vi "Defect Buddy.vi"() -> ()   [LabVIEW 2010]
uses:
  <vilib>/addons/database/Connection.llb/Conn ObjectReference.ctl
  <vilib>/addons/database/_DB Variant To Data/Database Variant To Data.xnode
  <vilib>/addons/database/Connection.llb/DB Tools Open Connec (Path).vi
  <vilib>/addons/database/Connection.llb/Conn Execute.vi
  <vilib>/addons/database/Recordset.llb/Rec Fetch Recordset Data (R).vi
  <vilib>/addons/database/Recordset.llb/Rec Destroy - Connection.vi
  <vilib>/Utility/file.llb/Write To Spreadsheet File (string).vi
  <vilib>/addons/database/NI_Database_API.lvlib
  <vilib>/picture/3D Picture Control/NI_3D Picture Control.lvlib
panel:
  out "Plot Names":string[][](array[string])
  out "Separate Defects":cluster{i32, i32}[](array[cluster])
  in  "Bound Pairs":T1(array[cluster])
  out "Array 2":T2(array[cluster])
  out "Array":string[][](array[string])
  out "spreadsheet string":string
  in  "Volumes":dbl[](array[numeric])=[5230.5515143, 4360.60278, 2309.371815, 7792.576126]
  in  "Markov-Payne Correction":bool=TRUE
  out "Loaded Structure":T3={"Structure Name"="Batch6_3+111 Quasi-Bulk", "Lattice vector a"=[9.1641, 0.0, 0.0], "Lattice vector b"=[0.0, 7.93635, 0.0], "Lattice vector c"=[0.0, 0.0, 53.7091], "Atoms Array"=[{"Atom Name"="", "Positions (Direct)"=[[0.036896, 0.129554, 0.035254], [0.536896, 0.129554, 0.035254], [0.286896, 0.629554, 0.035254], [0.786896, 0.629554, 0.035254], [0.285415, 0.295133, 0.107673], [0.785415, 0.295133, 0.107673], [0.035415, 0.795133, 0.107673], [0.535415, 0.795133, 0.107673], [0.033615, 0.463308, 0.180101], [0.533615, 0.463308, 0.180101], [0.283615, 0.963308, 0.180101], [0.783615, 0.963308, 0.180101], [0.030844, 0.131453, 0.252535], [0.530844, 0.131453, 0.252535], [0.280844, 0.631453, 0.252535], [0.780844, 0.631453, 0.252535], [0.278379, 0.302058, 0.324923], [0.778379, 0.302058, 0.324923], [0.028379, 0.802058, 0.324923], [0.528379, 0.802058, 0.324923], [0.031198, 0.471844, 0.397363], [0.531198, 0.471844, 0.397363], [0.281198, 0.971844, 0.397363], [0.781198, 0.971844, 0.397363], [0.03247, 0.140643, 0.469814], [0.53247, 0.140643, 0.469814], [0.28247, 0.640643, 0.469814], [0.78247, 0.640643, 0.469814], [0.284308, 0.303948, 0.542263], [0.784308, 0.303948, 0.542263], [0.034308, 0.803948, 0.542263], [0.534308, 0.803948, 0.542263], [0.035944, 0.468219, 0.614701], [0.535944, 0.468219, 0.614701], [0.285944, 0.968219, 0.614701], [0.785944, 0.968219, 0.614701], [0.037813, 0.131858, 0.687216], [0.537813, 0.131858, 0.687216], [0.787813, 0.631858, 0.687216], [0.287813, 0.631858, 0.687216], [0.038238, 0.463759, 0.759817], [0.538238, 0.463759, 0.759817], [0.288238, 0.963758, 0.759817], [0.788238, 0.963758, 0.759817], [0.038639, 0.130134, 0.831025], [0.538639, 0.130134, 0.831025], [0.288639, 0.630134, 0.831025], [0.788639, 0.630134, 0.831025], [0.285712, 0.295024, 0.89873], [0.785712, 0.295024, 0.89873], [0.035712, 0.795024, 0.89873], [0.535712, 0.795024, 0.89873], [0.032596, 0.464879, 0.966384], [0.532596, 0.464879, 0.966384], [0.282596, 0.964879, 0.966384], [0.782596, 0.964879, 0.966384]], "Positions (Cartesian)"=[[0.33811863359999994, 1.0281858879, 1.8934606114], [4.9201686336, 1.0281858879, 1.8934606114], [2.6291436335999996, 4.9963608879, 1.8934606114], [7.2111936336, 4.9963608879, 1.8934606114], [2.6155716014999997, 2.34227878455, 5.7830199243000004], [7.197621601499999, 2.34227878455, 5.7830199243000004], [0.3245466015, 6.31045378455, 5.7830199243000004], [4.9065966014999995, 6.31045378455, 5.7830199243000004], [0.30805122149999997, 3.6769744458, 9.673062619100001], [4.890101221499999, 3.6769744458, 9.673062619100001], [2.5990762215, 7.6451494458, 9.673062619100001], [7.1811262215, 7.6451494458, 9.673062619100001], [0.2826575004, 1.04325701655, 13.5634275685], [4.8647075004, 1.04325701655, 13.5634275685], [2.5736825004, 5.011432016550001, 13.5634275685], [7.155732500399999, 5.011432016550001, 13.5634275685], [2.5510929938999998, 2.3972380083, 17.4513218993], [7.1331429939, 2.3972380083, 17.4513218993], [0.2600679939, 6.3654130083, 17.4513218993], [4.8421179939000005, 6.3654130083, 17.4513218993], [0.28590159179999997, 3.7447191294, 21.3420091033], [4.867951591799999, 3.7447191294, 21.3420091033], [2.5769265918, 7.7128941294, 21.3420091033], [7.158976591799999, 7.7128941294, 21.3420091033], [0.29755832699999996, 1.11619207305, 25.2332871074], [4.879608327, 1.11619207305, 25.2332871074], [2.588583327, 5.08436707305, 25.2332871074], [7.170633327, 5.08436707305, 25.2332871074], [2.6054269428, 2.4122377098, 29.124457693300002], [7.1874769428, 2.4122377098, 29.124457693300002], [0.31440194279999994, 6.3804127098, 29.124457693300002], [4.8964519428, 6.3804127098, 29.124457693300002], [0.32939441039999995, 3.71594986065, 33.0150374791], [4.9114444104, 3.71594986065, 33.0150374791], [2.6204194104, 7.684124860650001, 33.0150374791], [7.202469410399999, 7.684124860650001, 33.0150374791], [0.3465221133, 1.0464712383, 36.909752865600005], [4.9285721133, 1.0464712383, 36.909752865600005], [7.2195971133, 5.0146462383, 36.909752865600005], [2.6375471132999997, 5.0146462383, 36.909752865600005], [0.3504168558, 3.6805537396499997, 40.809087234699994], [4.9324668557999995, 3.6805537396499997, 40.809087234699994], [2.6414418557999997, 7.6487208033, 40.809087234699994], [7.2234918558, 7.6487208033, 40.809087234699994], [0.35409165989999997, 1.0327889709, 44.6336048275], [4.9361416599, 1.0327889709, 44.6336048275], [2.6451166599, 5.0009639709, 44.6336048275], [7.227166659899999, 5.0009639709, 44.6336048275], [2.6182933392, 2.3414137224, 48.269979443000004], [7.200343339199999, 2.3414137224, 48.269979443000004], [0.3272683392, 6.3095887224, 48.269979443000004], [4.9093183391999995, 6.3095887224, 48.269979443000004], [0.29871300359999997, 3.6894424516499997, 51.9036148944], [4.880763003599999, 3.6894424516499997, 51.9036148944], [2.5897380036, 7.65761745165, 51.9036148944], [7.171788003599999, 7.65761745165, 51.9036148944]]}, {"Atom Name"="", "Positions (Direct)"=[[0.286795, 0.296109, 0.054458], [0.786795, 0.296109, 0.054458], [0.036795, 0.796109, 0.054458], [0.536795, 0.796109, 0.054458], [0.035258, 0.462031, 0.126878], [0.535258, 0.462031, 0.126878], [0.285258, 0.962031, 0.126878], [0.785258, 0.962031, 0.126878], [0.033445, 0.130094, 0.199309], [0.533445, 0.130094, 0.199309], [0.283445, 0.630094, 0.199309], [0.783445, 0.630094, 0.199309], [0.280766, 0.298203, 0.27171], [0.780766, 0.298203, 0.27171], [0.030766, 0.798203, 0.27171], [0.530766, 0.798203, 0.27171], [0.028505, 0.468822, 0.344121], [0.528505, 0.468822, 0.344121], [0.278505, 0.968822, 0.344121], [0.778505, 0.968822, 0.344121], [0.03126, 0.138635, 0.416572], [0.53126, 0.138635, 0.416572], [0.28126, 0.638635, 0.416572], [0.78126, 0.638635, 0.416572], [0.282556, 0.307128, 0.489026], [0.782556, 0.307128, 0.489026], [0.032556, 0.807128, 0.489026], [0.532556, 0.807128, 0.489026], [0.034374, 0.470438, 0.56147], [0.534374, 0.470438, 0.56147], [0.284374, 0.970438, 0.56147], [0.784374, 0.970438, 0.56147], [0.035964, 0.134698, 0.633895], [0.535964, 0.134698, 0.633895], [0.285964, 0.634698, 0.633895], [0.785964, 0.634698, 0.633895], [0.037794, 0.465111, 0.706493], [0.537794, 0.465111, 0.706493], [0.787794, 0.965111, 0.706493], [0.287794, 0.965111, 0.706493], [0.038181, 0.130274, 0.779081], [0.538181, 0.130274, 0.779081], [0.288181, 0.630273, 0.779081], [0.788181, 0.630273, 0.779081], [0.288548, 0.296604, 0.847022], [0.788548, 0.296604, 0.847022], [0.038548, 0.796604, 0.847022], [0.538548, 0.796604, 0.847022], [0.035661, 0.461866, 0.914714], [0.535661, 0.461866, 0.914714], [0.285661, 0.961866, 0.914714], [0.785661, 0.961866, 0.914714], [0.032517, 0.131341, 0.982331], [0.532517, 0.131341, 0.982331], [0.282517, 0.631341, 0.982331], [0.782517, 0.631341, 0.982331]], "Positions (Cartesian)"=[[2.6282180595, 2.35002466215, 2.9248901678], [7.2102680595, 2.35002466215, 2.9248901678], [0.3371930595, 6.31819966215, 2.9248901678], [4.9192430595, 6.31819966215, 2.9248901678], [0.32310783779999996, 3.66683972685, 6.814503189799999], [4.9051578378, 3.66683972685, 6.814503189799999], [2.6141328378, 7.63501472685, 6.814503189799999], [7.1961828377999995, 7.63501472685, 6.814503189799999], [0.3064933245, 1.0324715168999998, 10.704707011899998], [4.8885433245, 1.0324715168999998, 10.704707011899998], [2.5975183244999998, 5.000646516900001, 10.704707011899998], [7.179568324499999, 5.000646516900001, 10.704707011899998], [2.5729677006, 2.36664337905, 14.593299561], [7.155017700599999, 2.36664337905, 14.593299561], [0.2819427006, 6.33481837905, 14.593299561], [4.863992700599999, 6.33481837905, 14.593299561], [0.2612226705, 3.7207354797, 18.4824292011], [4.843272670499999, 3.7207354797, 18.4824292011], [2.5522476705, 7.6889104797, 18.4824292011], [7.1342976705, 7.6889104797, 18.4824292011], [0.286469766, 1.1002558822500002, 22.3737072052], [4.8685197659999995, 1.1002558822500002, 22.3737072052], [2.577494766, 5.0684308822499995, 22.3737072052], [7.159544765999999, 5.0684308822499995, 22.3737072052], [2.5893714396, 2.4374753028000002, 26.2651463366], [7.1714214396, 2.4374753028000002, 26.2651463366], [0.2983464396, 6.4056503028, 26.2651463366], [4.8803964396, 6.4056503028, 26.2651463366], [0.3150067734, 3.7335606213, 30.156048377], [4.8970567734, 3.7335606213, 30.156048377], [2.6060317734, 7.7017356213, 30.156048377], [7.1880817733999995, 7.7017356213, 30.156048377], [0.3295776924, 1.0690104723, 34.045929944499996], [4.9116276924, 1.0690104723, 34.045929944499996], [2.6206026924, 5.0371854723, 34.045929944499996], [7.202652692399999, 5.0371854723, 34.045929944499996], [0.3463479954, 3.69128368485, 37.9451031863], [4.928397995399999, 3.69128368485, 37.9451031863], [7.2194229953999995, 7.659458684850001, 37.9451031863], [2.6373729954, 7.659458684850001, 37.9451031863], [0.34989450209999995, 1.0339000599000001, 41.843739337100004], [4.9319445020999995, 1.0339000599000001, 41.843739337100004], [2.6409195021, 5.00206712355, 41.843739337100004], [7.2229695021, 5.00206712355, 41.843739337100004], [2.6442827268, 2.3539531553999997, 45.4927893002], [7.2263327268, 2.3539531553999997, 45.4927893002], [0.35325772679999995, 6.3221281554, 45.4927893002], [4.9353077268, 6.3221281554, 45.4927893002], [0.3268009701, 3.6655302291, 49.1284656974], [4.9088509701000005, 3.6655302291, 49.1284656974], [2.6178259700999997, 7.6337052291, 49.1284656974], [7.1998759701, 7.6337052291, 49.1284656974], [0.29798903969999996, 1.04236814535, 52.760113912099996], [4.8800390397, 1.04236814535, 52.760113912099996], [2.5890140397, 5.010543145350001, 52.760113912099996], [7.1710640397, 5.010543145350001, 52.760113912099996]]}], "# of atoms"=112}
  out "Indicies":cluster{i32, i32}[](array[cluster])
  out "All Hosts and Defects":T4(array[cluster])
  out "Thermodynamic Fermi Level (eV)":dbl
  out "Defects to Bind":i32[](array[numeric])
  in  "Plot Binding Energy":bool
  in  "Calc Thermodynamic Fermi Level":bool
  in  "Thermodynamic Fermi Level":i32
  in  "Color Array Type":T5(ring)=enum."Contrasting Colors"
  in  "Show Charge Transitions":bool=TRUE
  out "connection reference":T6
  in  "Plots Tab":T7(tab)
  in  "Make Awesome Looking":bool
  out "Te Rich Limit":cluster{dbl[], dbl[]}[](graph)
  out "Cd Rich Limit":cluster{"appended array":dbl[], dbl[]}[](graph)
  in  "Chemical Potential":dbl(slide) scale=0.0..1.0
  in  "Chemical Potential 2":dbl(slide)=1.0 scale=0.0..1.0
  in  "Save as a table":bool
  out "Te Rich Limit 2":cluster{dbl[], dbl[]}[](graph)
  out "Cd Rich Limit 2":cluster{"appended array":dbl[], dbl[]}[](graph)
  in  "Chemical Potential 5":dbl(slide) scale=0.0..1.0
  in  "Chemical Potential 3":dbl(slide)=1.0 scale=0.0..1.0
  in  "Save as a table 2":bool
  in  "Binding Energy":bool
  in  "Formation Energy":bool
  in  "Bound Pairs List":i32[](listbox)
  in  "Assign Bound Calculation":bool
  in  "Seperate Defects":i32(listbox)
  in  "Set as seperate defects":bool
  out "Binding Energy":cluster{"Array":dbl[], dbl[]}[](graph)
  in  "Binding Energy Chem Pot":dbl(slide) scale=0.0..1.0
  out "Defect Energy Levels":cluster{dbl[], dbl[]}[](graph)
  in  "Buckets":string[][](array[combo])
  out "Atomic Structure":refnum<vi>(3d-picture)
  in  "Load in VESTA":bool
  in  "Atomic Structures":i32(listbox)
  in  "Options":cluster{"Border?":bool, "Bonds?":bool}
  in  "Atom Size":dbl=0.75
  in  "Plot Atomic Structure":bool
  in  "Scale":dbl(slide)=0.07482993197278912 scale=0.0..0.5
  in  "Setup Camera":bool
  out "Table Control":string[][](table)
  in  "Ignore Location":bool
  in  "Potential Re-alignment":bool
  out "Defects":T8(array[cluster])
  out "Base Object":refnum<vi>
  in  "VBM":dbl=1.79581
  in  "Ignore Incomplete":bool
  in  "Pure Structures with defects":i32[](listbox)
  in  "Related Defects":i32[](listbox)
  in  "UDL":path=path "D:/Ab-initio/VASP Calcs/VASP DB.udl"
  # "Cd Rich"
  # "Te Rich"
  # "Cd Rich"
  # "Te Rich"
  # "p-type"
  # "n-type"
  # "p-type"
  # "n-type"
  # "Cd Rich"
  # "Te Rich"
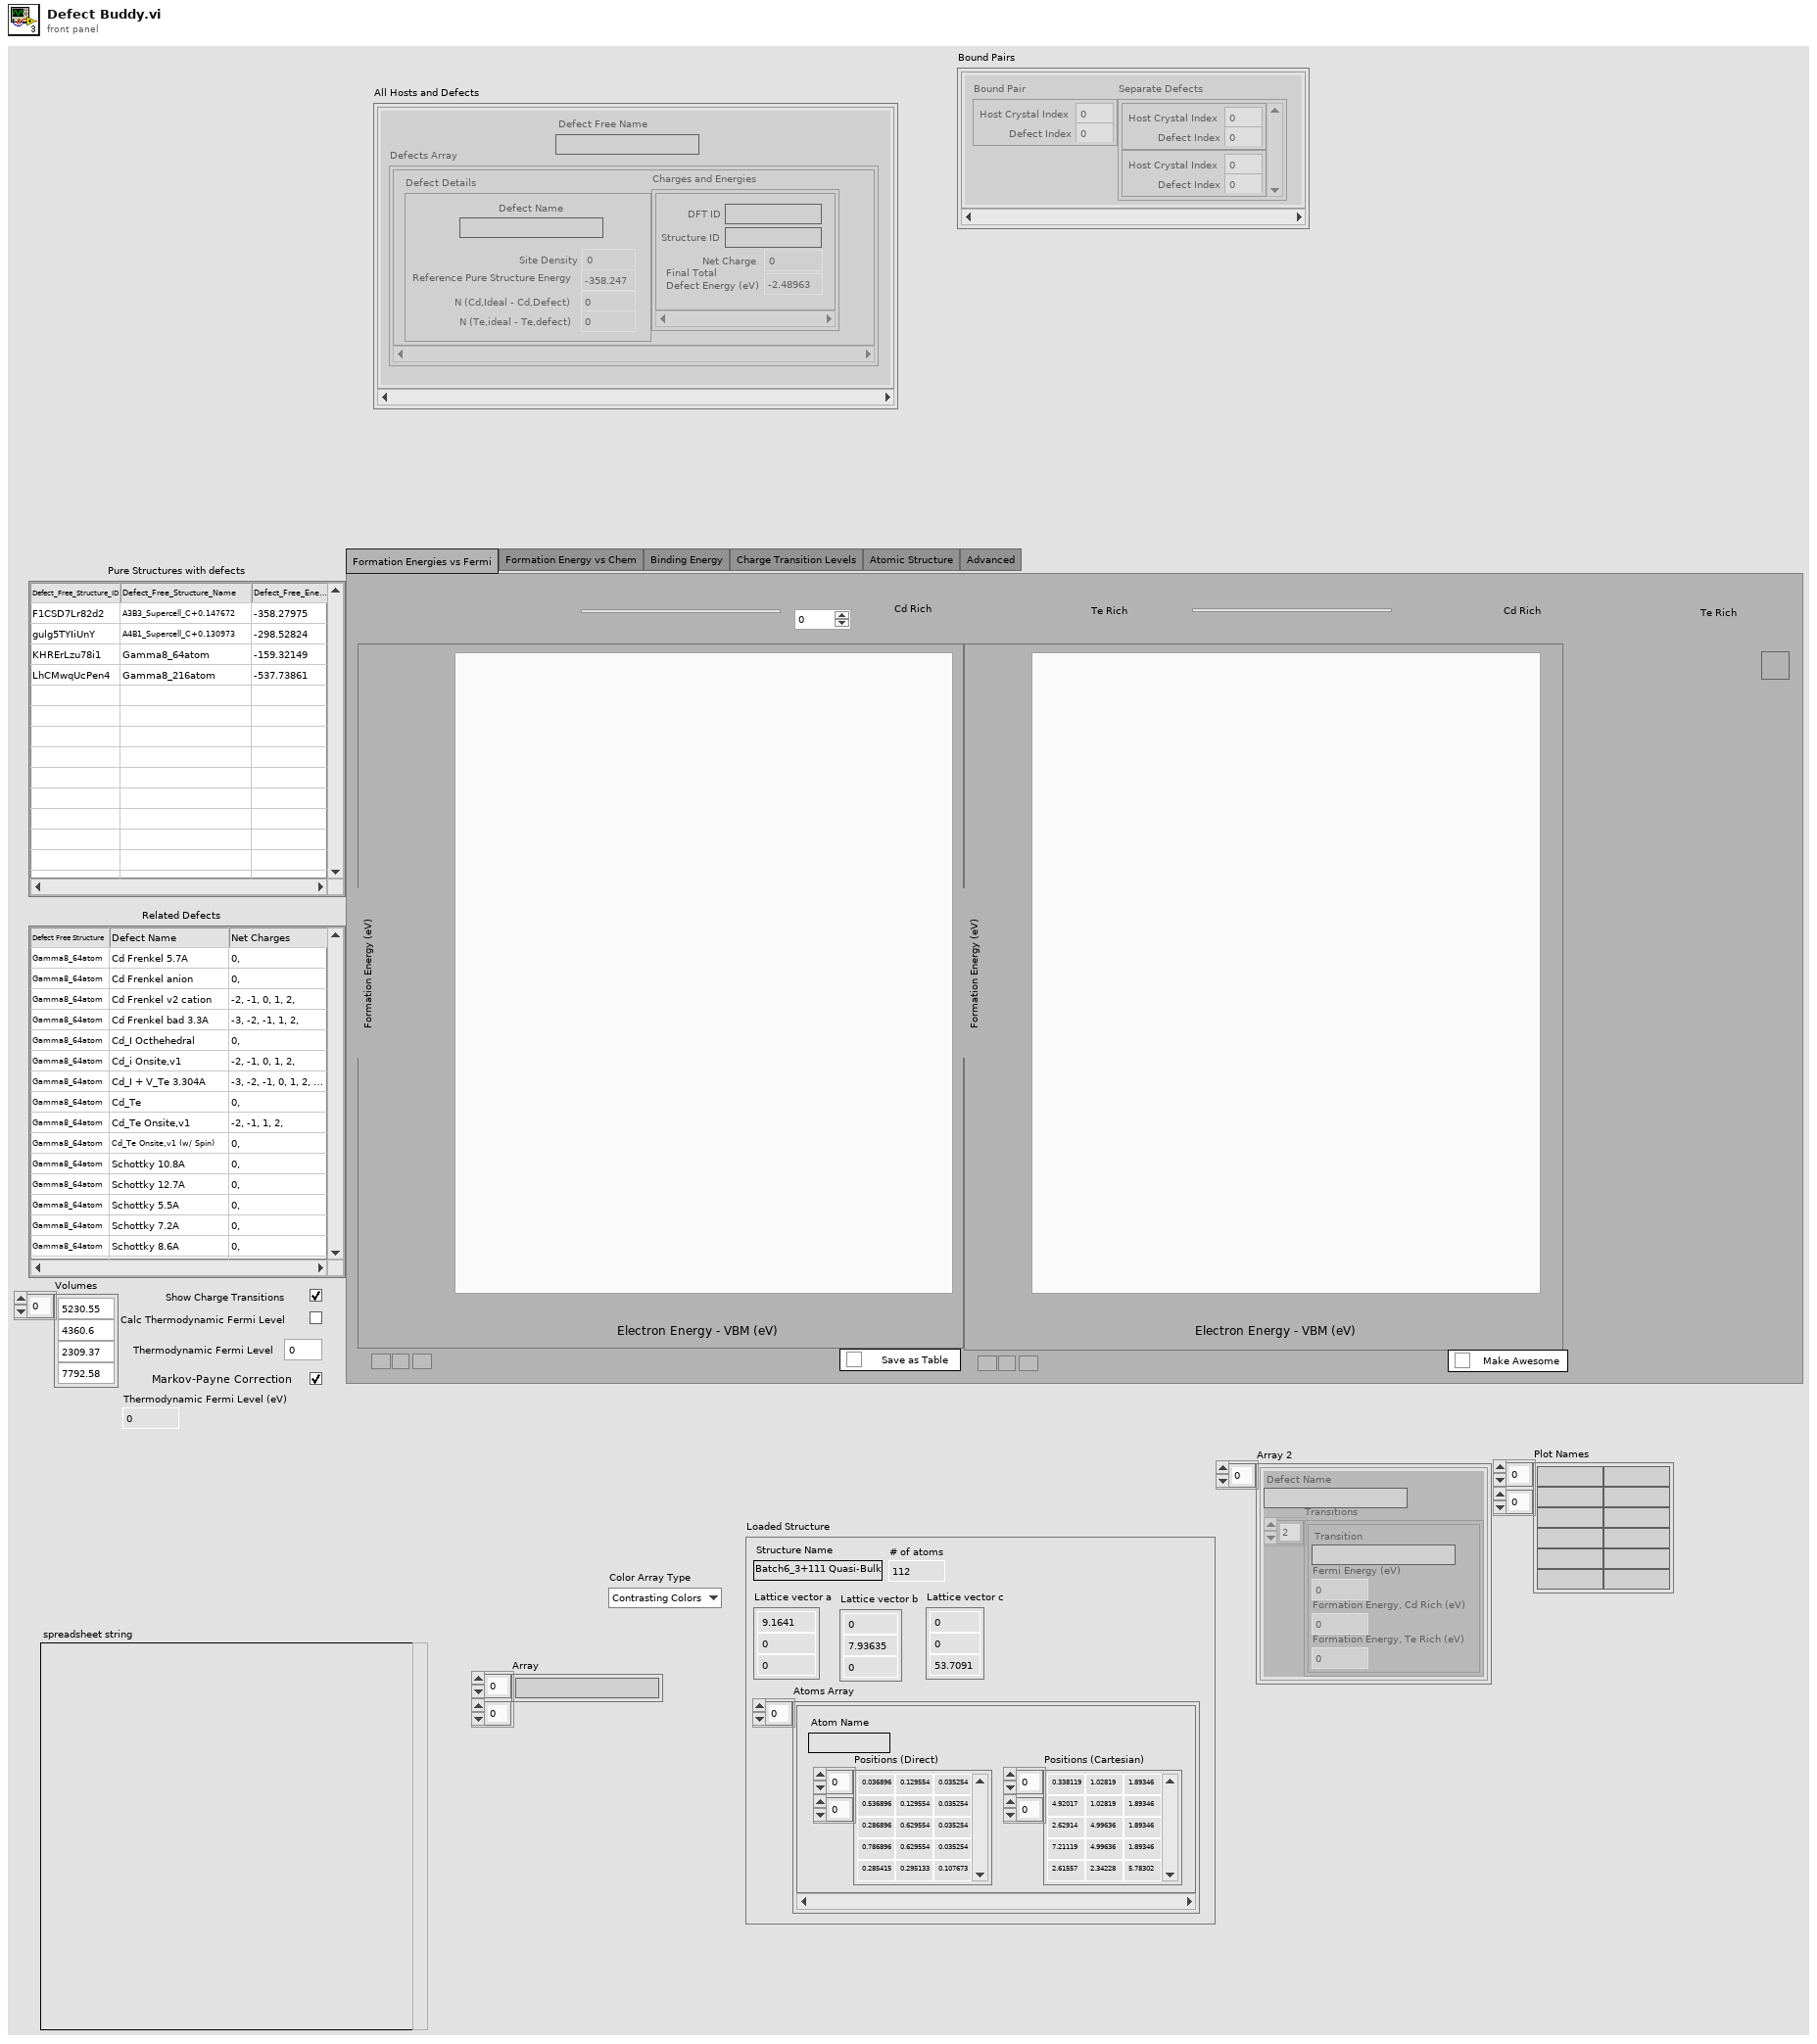
[diagram p1: front panel]
types:
  T1 = cluster{"Bound Pair":cluster{"Host Crystal Index":i32, "Defect Index":i32}, "Separate Defects":cluster{"Host Crystal Index":i32, "Defect Index":i32}[]}[]
  T2 = cluster{"Defect Name":string, "Transitions":cluster{"Transition":string, "Fermi Energy (eV)":dbl, "Formation Energy, Cd Rich (eV)":dbl, "Formation Energy, Te Rich (eV)":dbl}[]}[]
  T3 = cluster{"Structure Name":string, "Lattice vector a":dbl[], "Lattice vector b":dbl[], "Lattice vector c":dbl[], "Atoms Array":cluster{"Atom Name":string, "Positions (Direct)":dbl[][], "Positions (Cartesian)":dbl[][]}[], "# of atoms":i32}
  T4 = cluster{"Defect Free Name":string, "Defects Array":cluster{"Defect Details":cluster{"Defect Name":string, "Site Density":dbl, "Reference Pure Structure Energy":dbl, "N (Cd,Ideal - Cd,Defect)":i32, "N (Te,ideal - Te,defect)":i32}, "Charges and Energies":cluster{"DFT ID":string, "Structure ID":string, "Net Charge":i32, "Final Total \nDefect Energy (eV)":dbl}[]}[]}[]
  T5 = enum16{"Visible Spectrum", "Greyscale", "Contrasting Colors"}
  T6 = typedef "NI_Database_API.lvlib/Conn ObjectReference.ctl" = refnum<k1>
  T7 = enum32{"Formation Energies vs Fermi", "Formation Energy vs Chem", "Binding Energy", "Charge Transition Levels", "Atomic Structure", "Advanced"}
  T8 = cluster{"Defect Details":cluster{"Defect Name":string, "Site Density":dbl, "Reference Pure Structure Energy":dbl, "N (Cd,Ideal - Cd,Defect)":i32, "N (Te,ideal - Te,defect)":i32}, "Charges and Energies":cluster{"Net Charge":i32, "Final Total \nDefect Energy (eV)":dbl}[]}[]
  T9 = typedef "NI_Database_API.lvlib/Rec ObjectReference.ctl" = refnum<k1>
  T10 = cluster{"Name":string, "Color":u32, "Style":u8, "Point Style":u8, "Name Visible":bool, "Allow Drag":bool, "Annotation Mode":u32, "Plot":i32, "Index":i32, "Position":cluster{"X":dbl, "Y":dbl}, "X Scale":u32, "Y Scale":u32, "Show Arrow":bool, "Lock Name":bool, "Plot Area":i32, "Label Offset":cluster{"X":dbl, "Y":dbl}}
  T11 = cluster{"Name":string, "Color":u32, "Style":u8, "Point Style":u8, "Name Visible":bool, "Allow Drag":bool, "Cursor Mode":u32, "Plot":i32, "Index":i32, "Position":cluster{"X":dbl, "Y":dbl}, "X Scale":u32, "Y Scale":u32, "Watch Plots":i32[], "Watch All Plots":bool, "Plot Area":i32, "Label Offset":cluster{"X":dbl, "Y":dbl}}
  T12 = cluster{"Defect Details":cluster{"Defect Name":string, "Site Density":dbl, "Reference Pure Structure Energy":dbl, "N (Cd,Ideal - Cd,Defect)":i32, "N (Te,ideal - Te,defect)":i32}, "Charges and Energies":cluster{"DFT ID":string, "Structure ID":string, "Net Charge":i32, "Final Total \nDefect Energy (eV)":dbl}[]}[]
  T13 = cluster{"Defect Name":string, "Site Density":dbl, "Reference Pure Structure Energy":dbl, "N (Cd,Ideal - Cd,Defect)":i32, "N (Te,ideal - Te,defect)":i32}
  T14 = cluster{"DFT ID":string, "Structure ID":string, "Net Charge":i32, "Final Total \nDefect Energy (eV)":dbl}[]
  T15 = cluster{string, "Defects Array":cluster{"Defect Details":cluster{"Defect Name":string, "Site Density":dbl, "Reference Pure Structure Energy":dbl, "N (Cd,Ideal - Cd,Defect)":i32, "N (Te,ideal - Te,defect)":i32}, "Charges and Energies":cluster{"DFT ID":string, "Structure ID":string, "Net Charge":i32, "Final Total \nDefect Energy (eV)":dbl}[]}[]}
  T16 = cluster{"Name":string, "Color":u32, "Style":u8, "Point Style":u8, "Name Visible":bool, "Allow Drag":bool, "Cursor Mode":u32, "Plot":i32, "Index":i32, "Position":cluster{"X":dbl, "Y":dbl}, "X Scale":u32, "Y Scale":u32, "Watch Plots":i32[], "Watch All Plots":bool, "Plot Area":i32, "Label Offset":cluster{"X":dbl, "Y":dbl}}[]
  T17 = cluster{"Name":string, "Color":u32, "Style":u8, "Point Style":u8, "Name Visible":bool, "Allow Drag":bool, "Annotation Mode":u32, "Plot":i32, "Index":i32, "Position":cluster{"X":dbl, "Y":dbl}, "X Scale":u32, "Y Scale":u32, "Show Arrow":bool, "Lock Name":bool, "Plot Area":i32, "Label Offset":cluster{"X":dbl, "Y":dbl}}[]
  T18 = cluster{"Defect Free Name":string, "Defects Array":cluster{"Defect Details":cluster{"Defect Name":string, "Site Density":dbl, "Reference Pure Structure Energy":dbl, "N (Cd,Ideal - Cd,Defect)":i32, "N (Te,ideal - Te,defect)":i32}, "Charges and Energies":cluster{"DFT ID":string, "Structure ID":string, "Net Charge":i32, "Final Total \nDefect Energy (eV)":dbl}[]}[]}
  T19 = cluster{"Defect Details":cluster{"Defect Name":string, "Site Density":dbl, "Reference Pure Structure Energy":dbl, "N (Cd,Ideal - Cd,Defect)":i32, "N (Te,ideal - Te,defect)":i32}, "Charges and Energies":cluster{"DFT ID":string, "Structure ID":string, "Net Charge":i32, "Final Total \nDefect Energy (eV)":dbl}[]}
  T20 = cluster{"Transition":string, "Fermi Energy (eV)":dbl, "Formation Energy, Cd Rich (eV)":dbl, "Formation Energy, Te Rich (eV)":dbl}[]
  T21 = cluster{"Defect Name":string, "Transitions":cluster{"Transition":string, "Fermi Energy (eV)":dbl, "Formation Energy, Cd Rich (eV)":dbl, "Formation Energy, Te Rich (eV)":dbl}[]}
  T22 = cluster{cluster{i32, i32}, "Separate Defects":cluster{i32, i32}[]}
  T23 = cluster{"Bound Pair":cluster{"Host Crystal Index":i32, "Defect Index":i32}, "Separate Defects":cluster{"Host Crystal Index":i32, "Defect Index":i32}[]}
  T24 = cluster{"Host Crystal Index":i32, "Defect Index":i32}
  T25 = cluster{"Host Crystal Index":i32, "Defect Index":i32}[]
  T26 = cluster{"Lattice vector b[0]":dbl, "Lattice vector b[1]":dbl, "Lattice vector b[2]":dbl}
  T27 = typedef "LVAnnotationListTypeDef.ctl" = cluster{"Name":string, "Color":u32, "Style":u8, "Point Style":u8, "Name Visible":bool, "Allow Drag":bool, "Annotation Mode":u32, "Plot":i32, "Index":i32, "Position":cluster{"X":dbl, "Y":dbl}, "X Scale":u32, "Y Scale":u32, "Show Arrow":bool, "Lock Name":bool, "Plot Area":i32, "Label Offset":cluster{"X":dbl, "Y":dbl}}[]
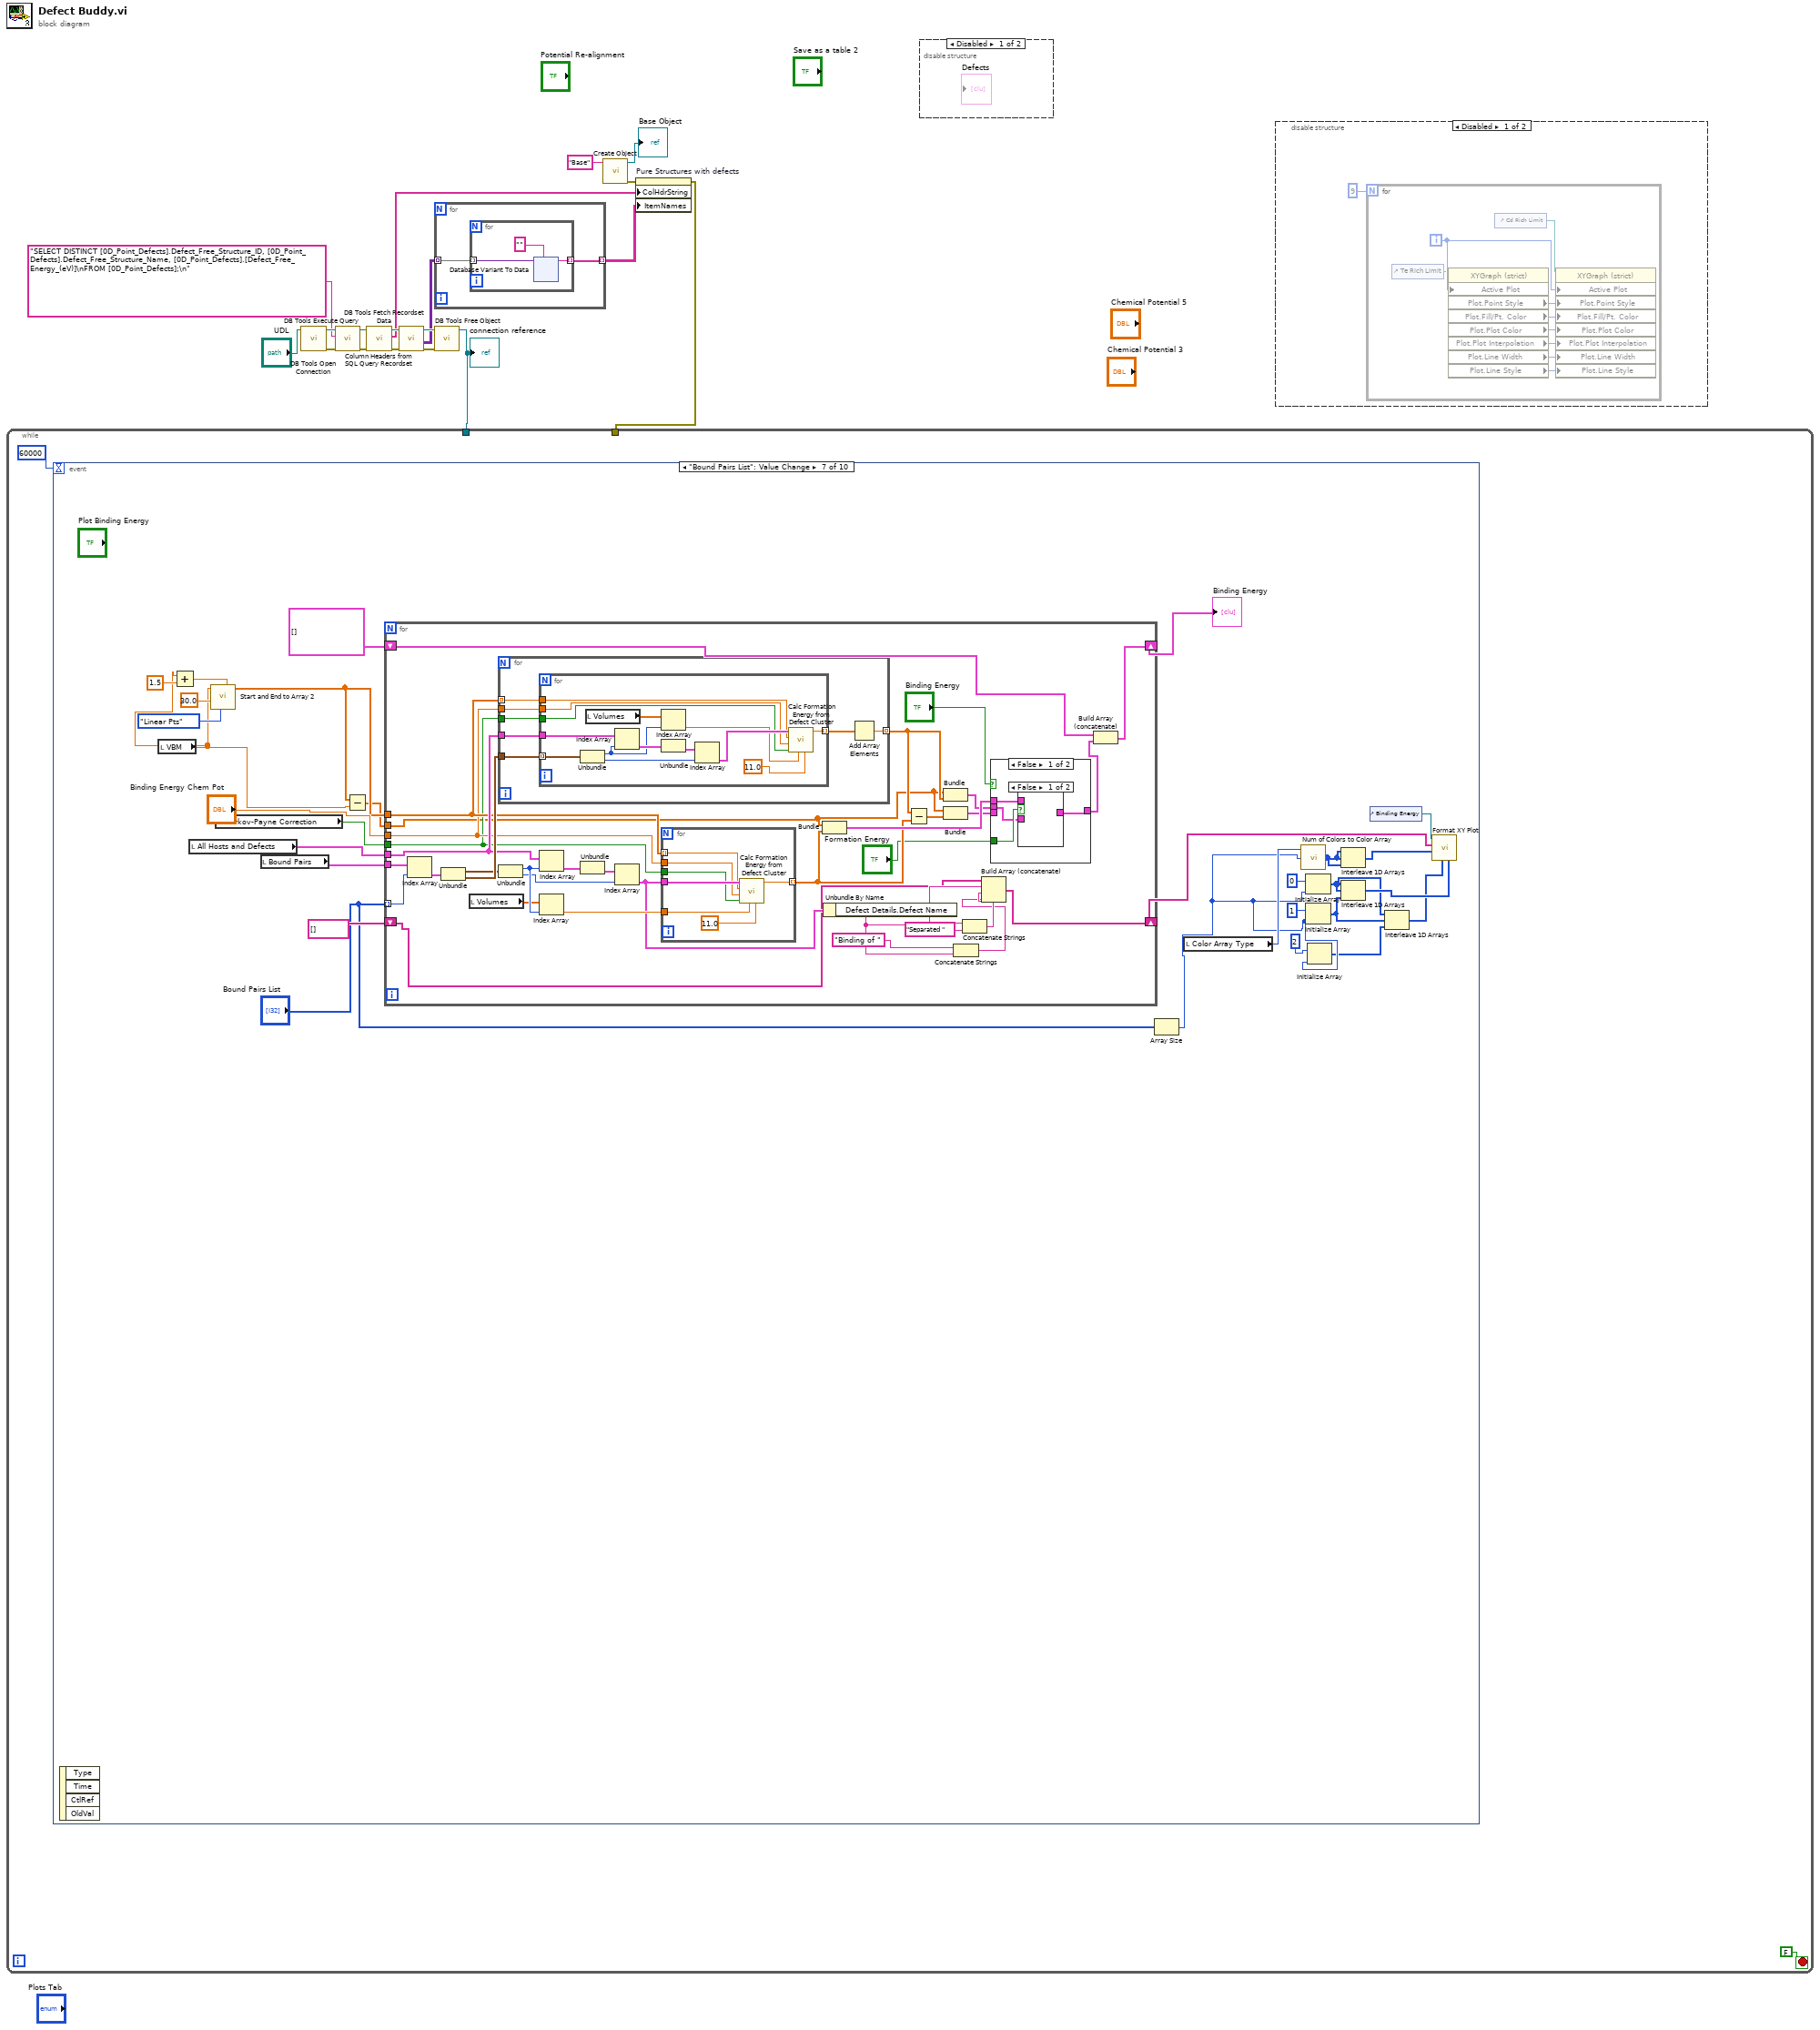
[diagram p0: block diagram]
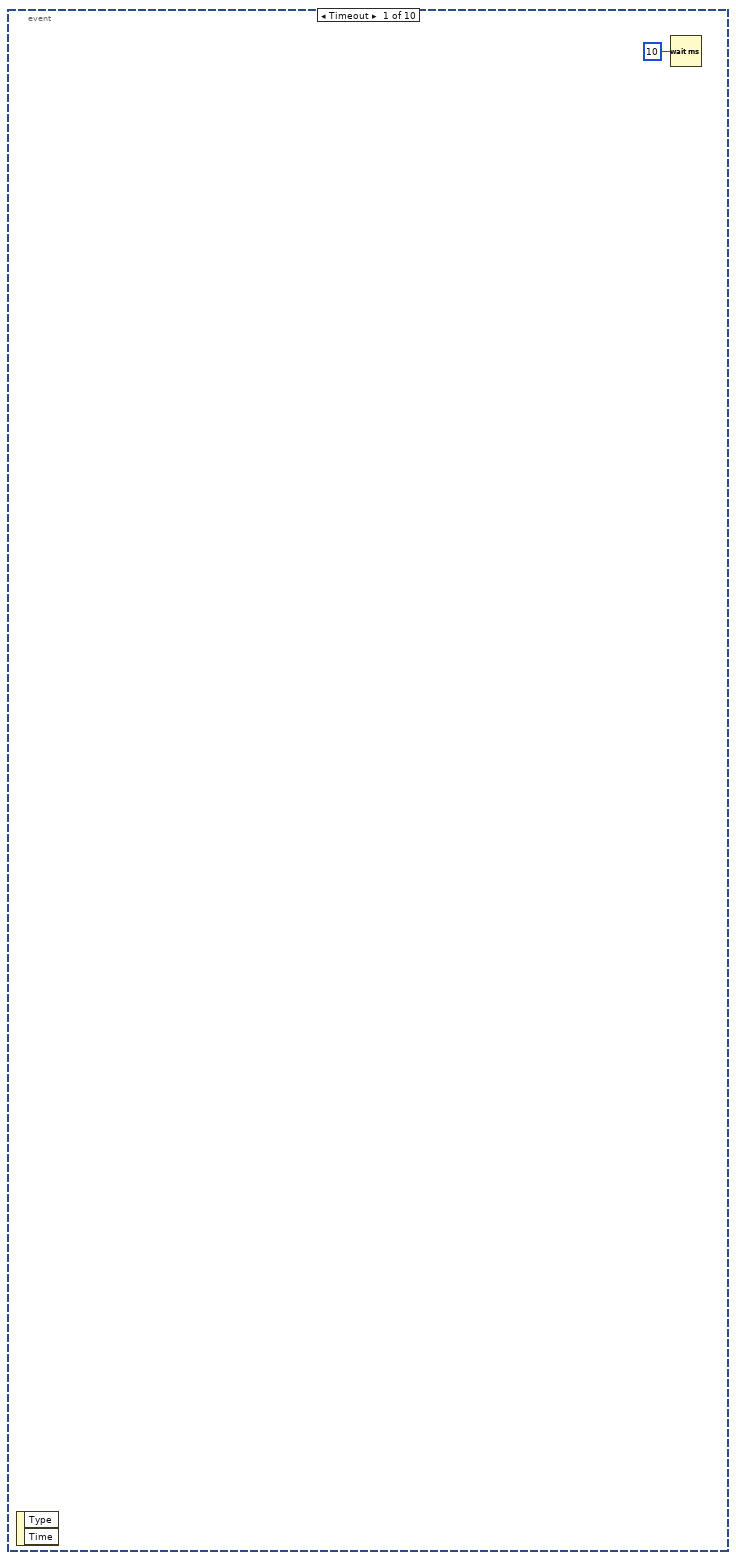
[diagram p4: hidden frame]
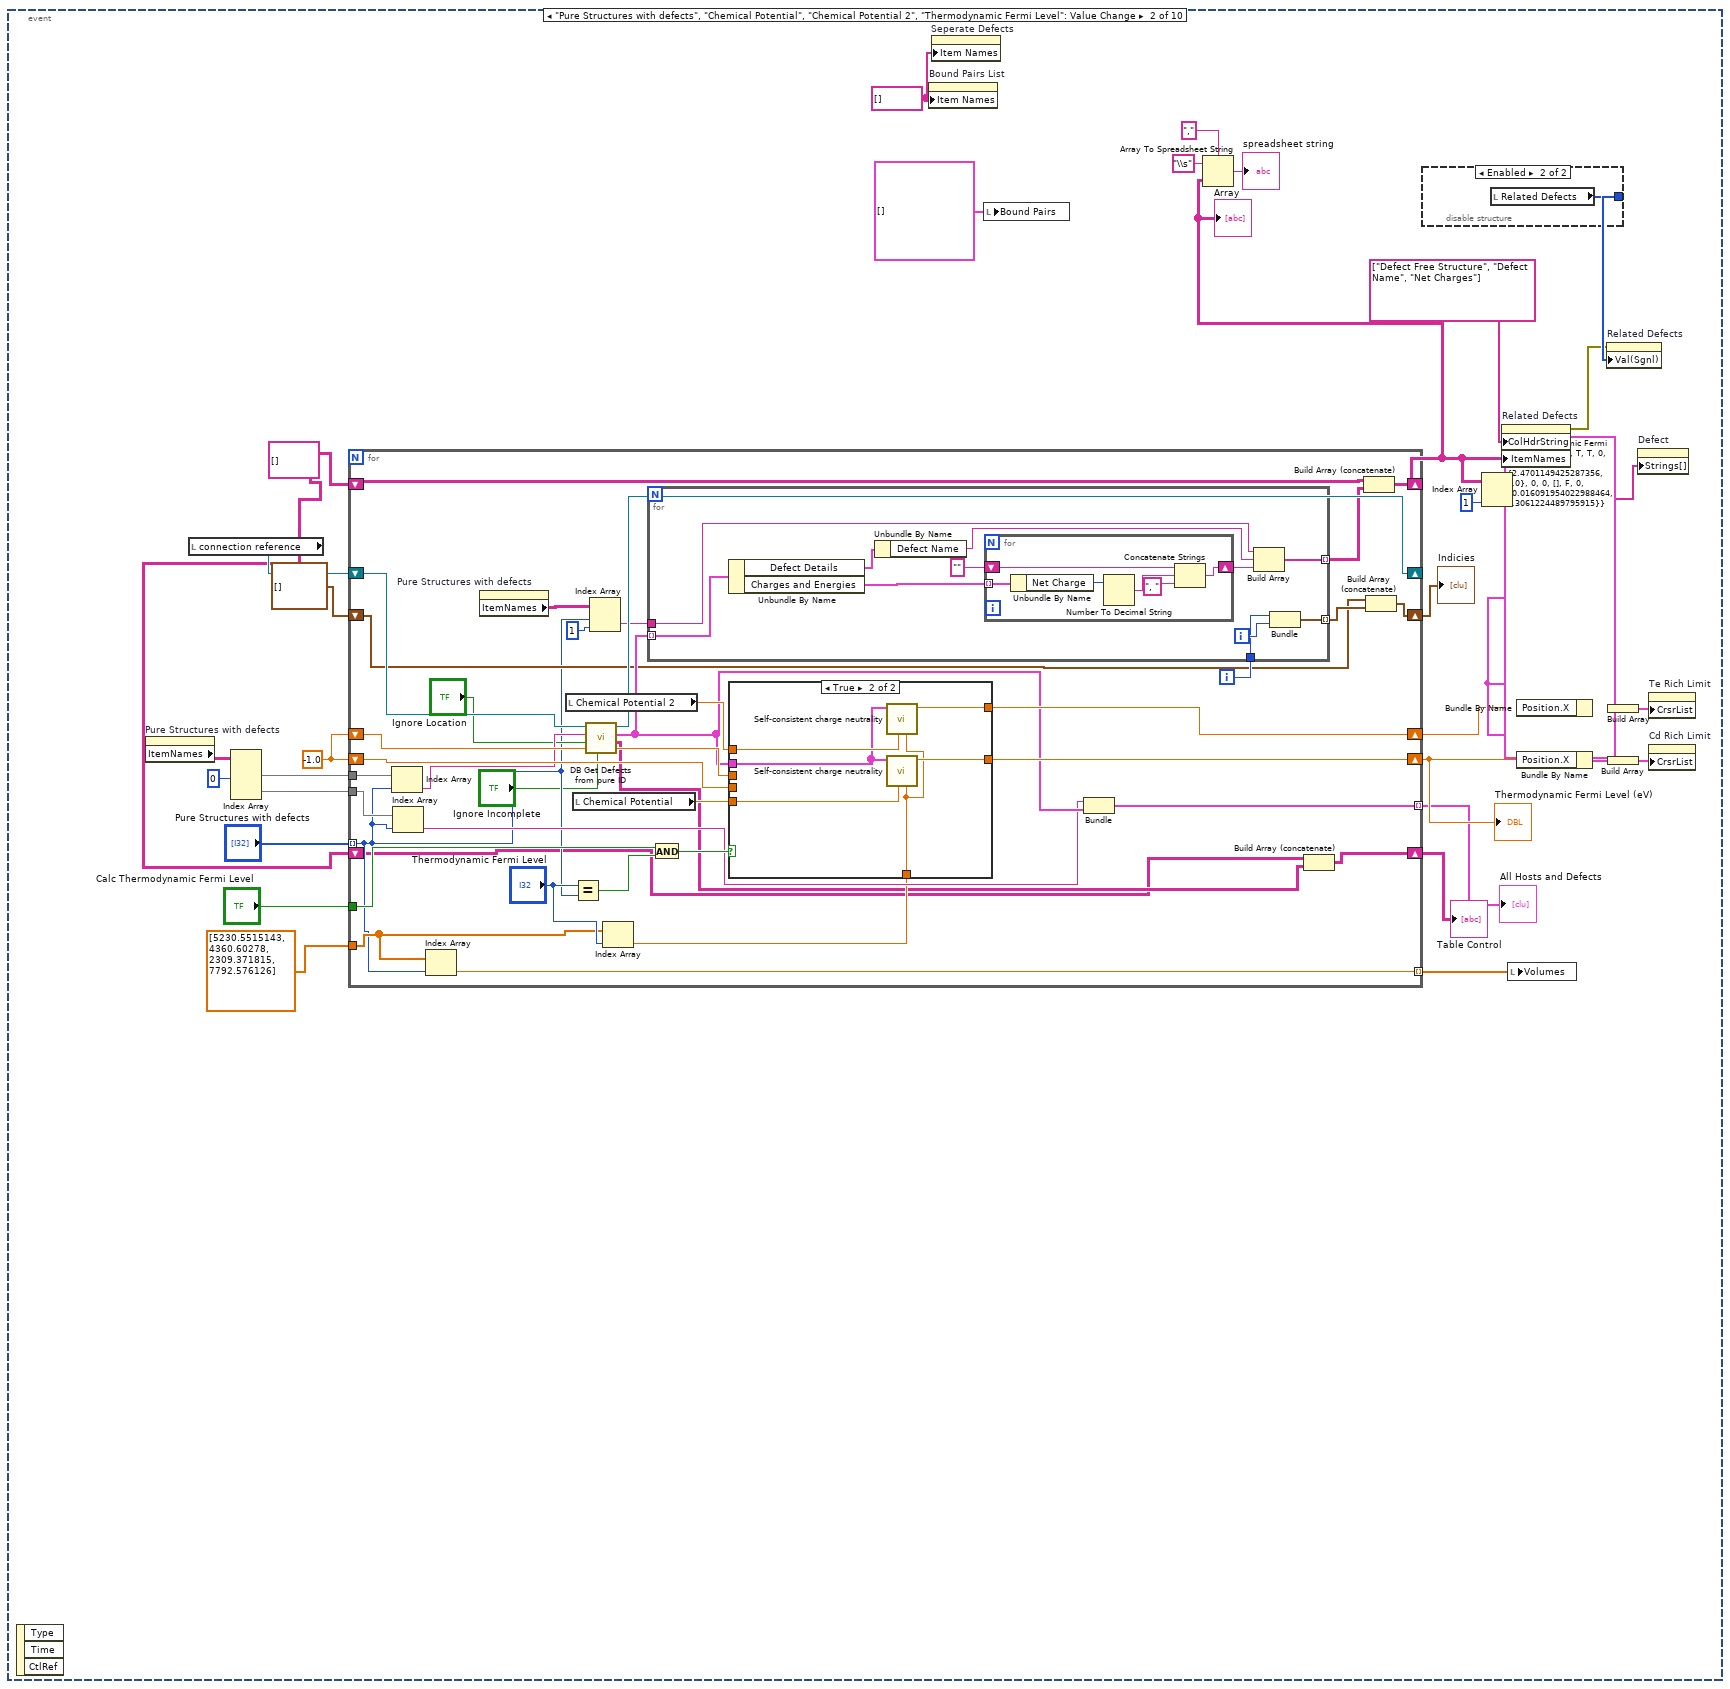
[diagram p5: hidden frame]
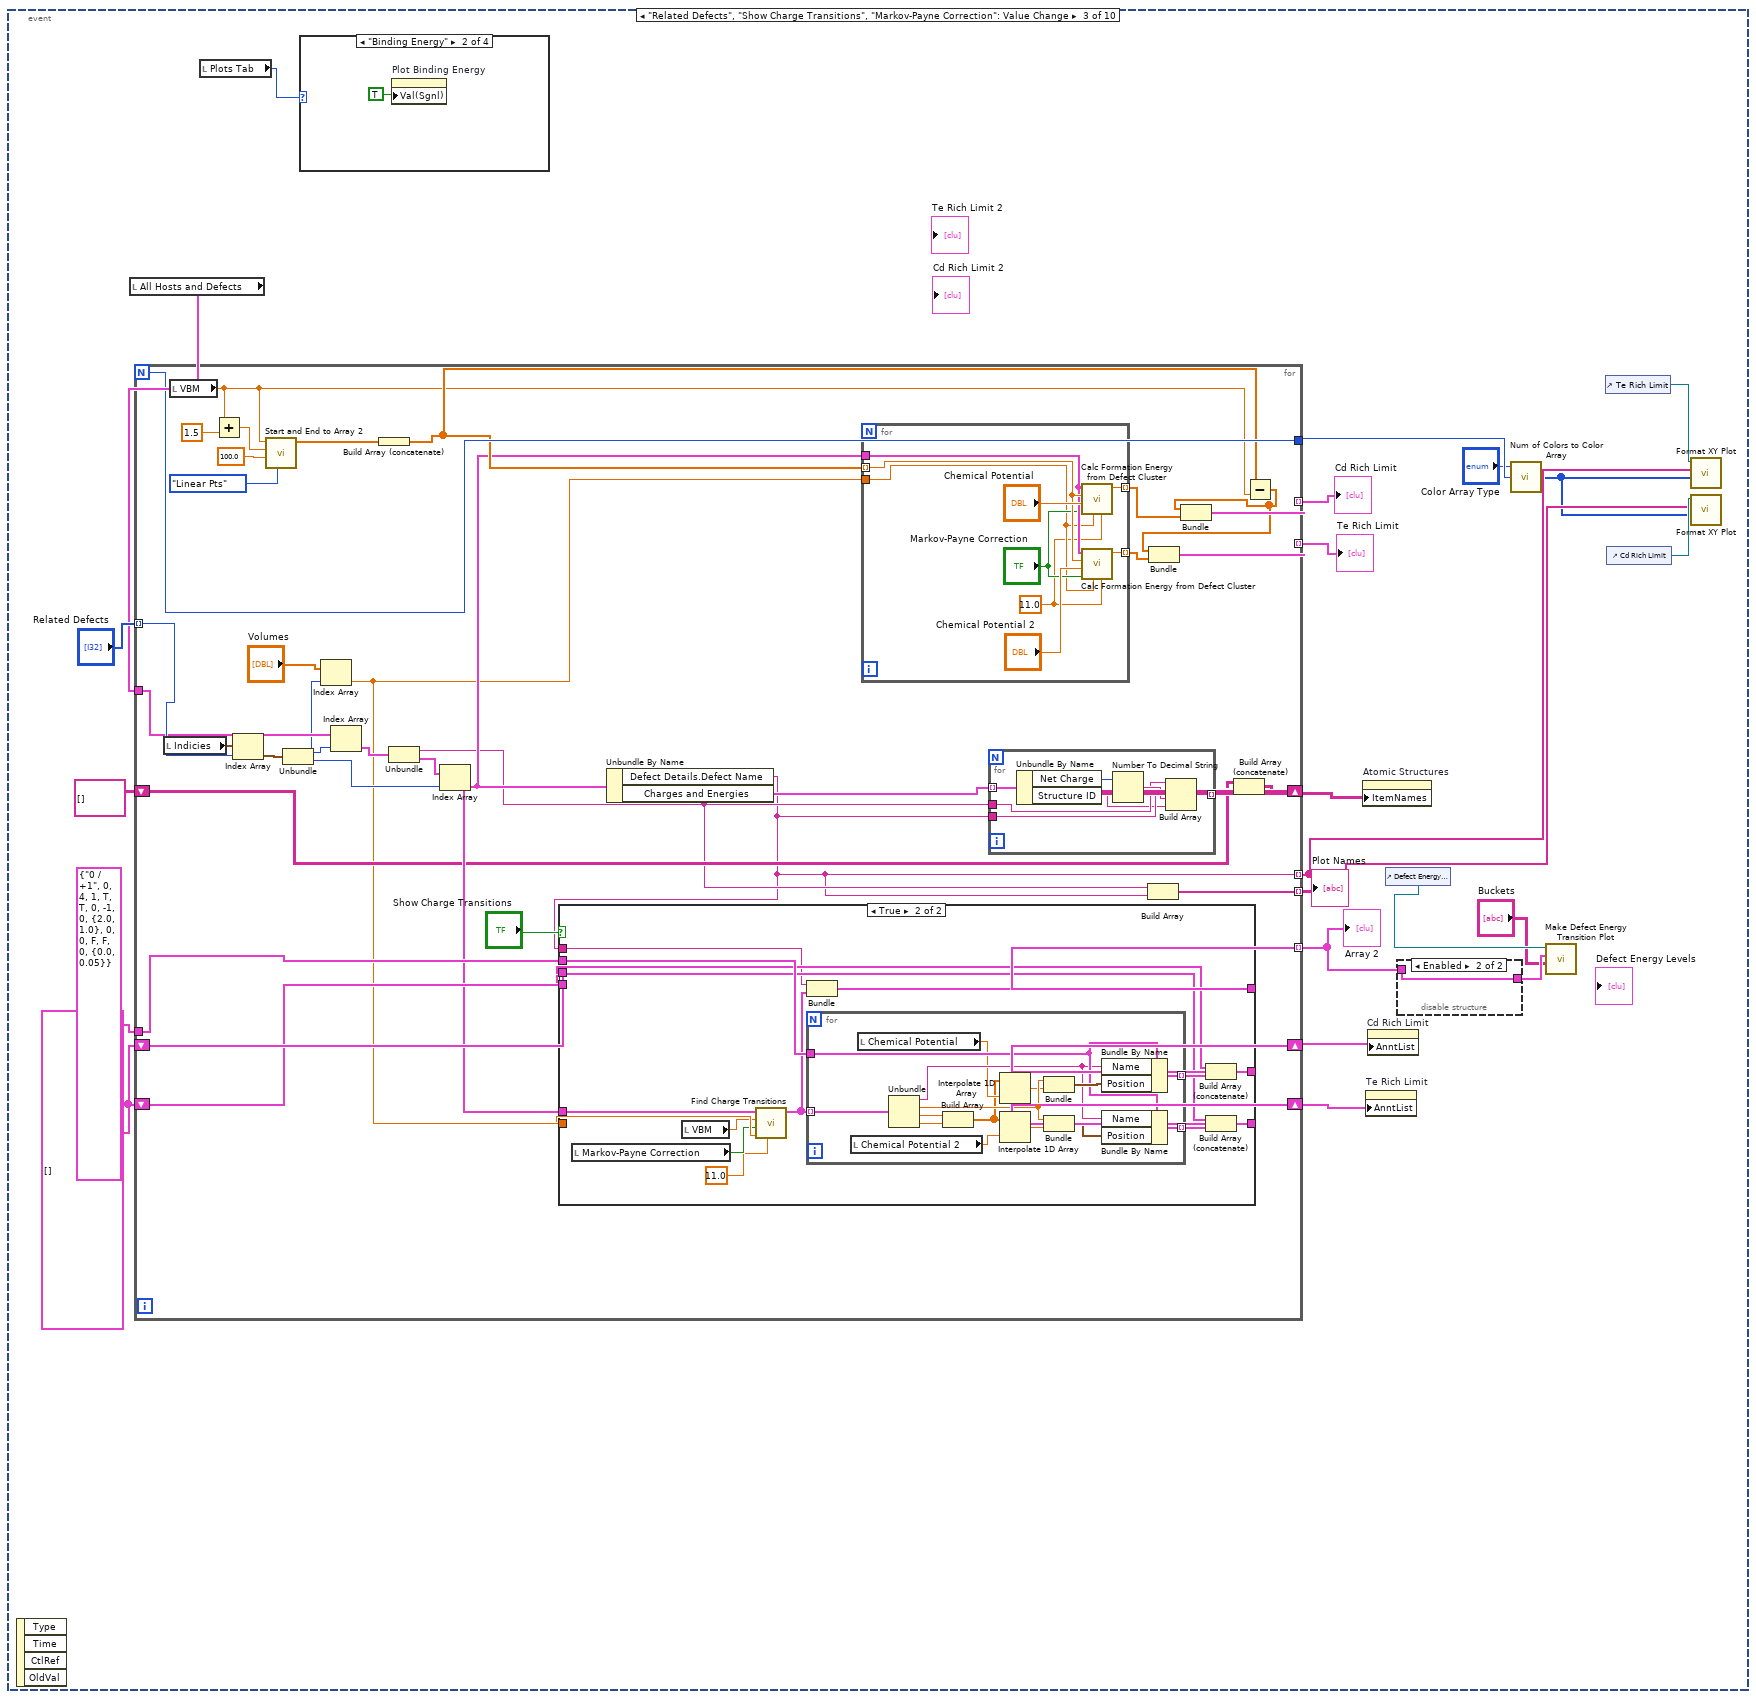
[diagram p8: hidden frame]
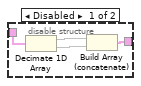
[diagram p9: hidden frame]
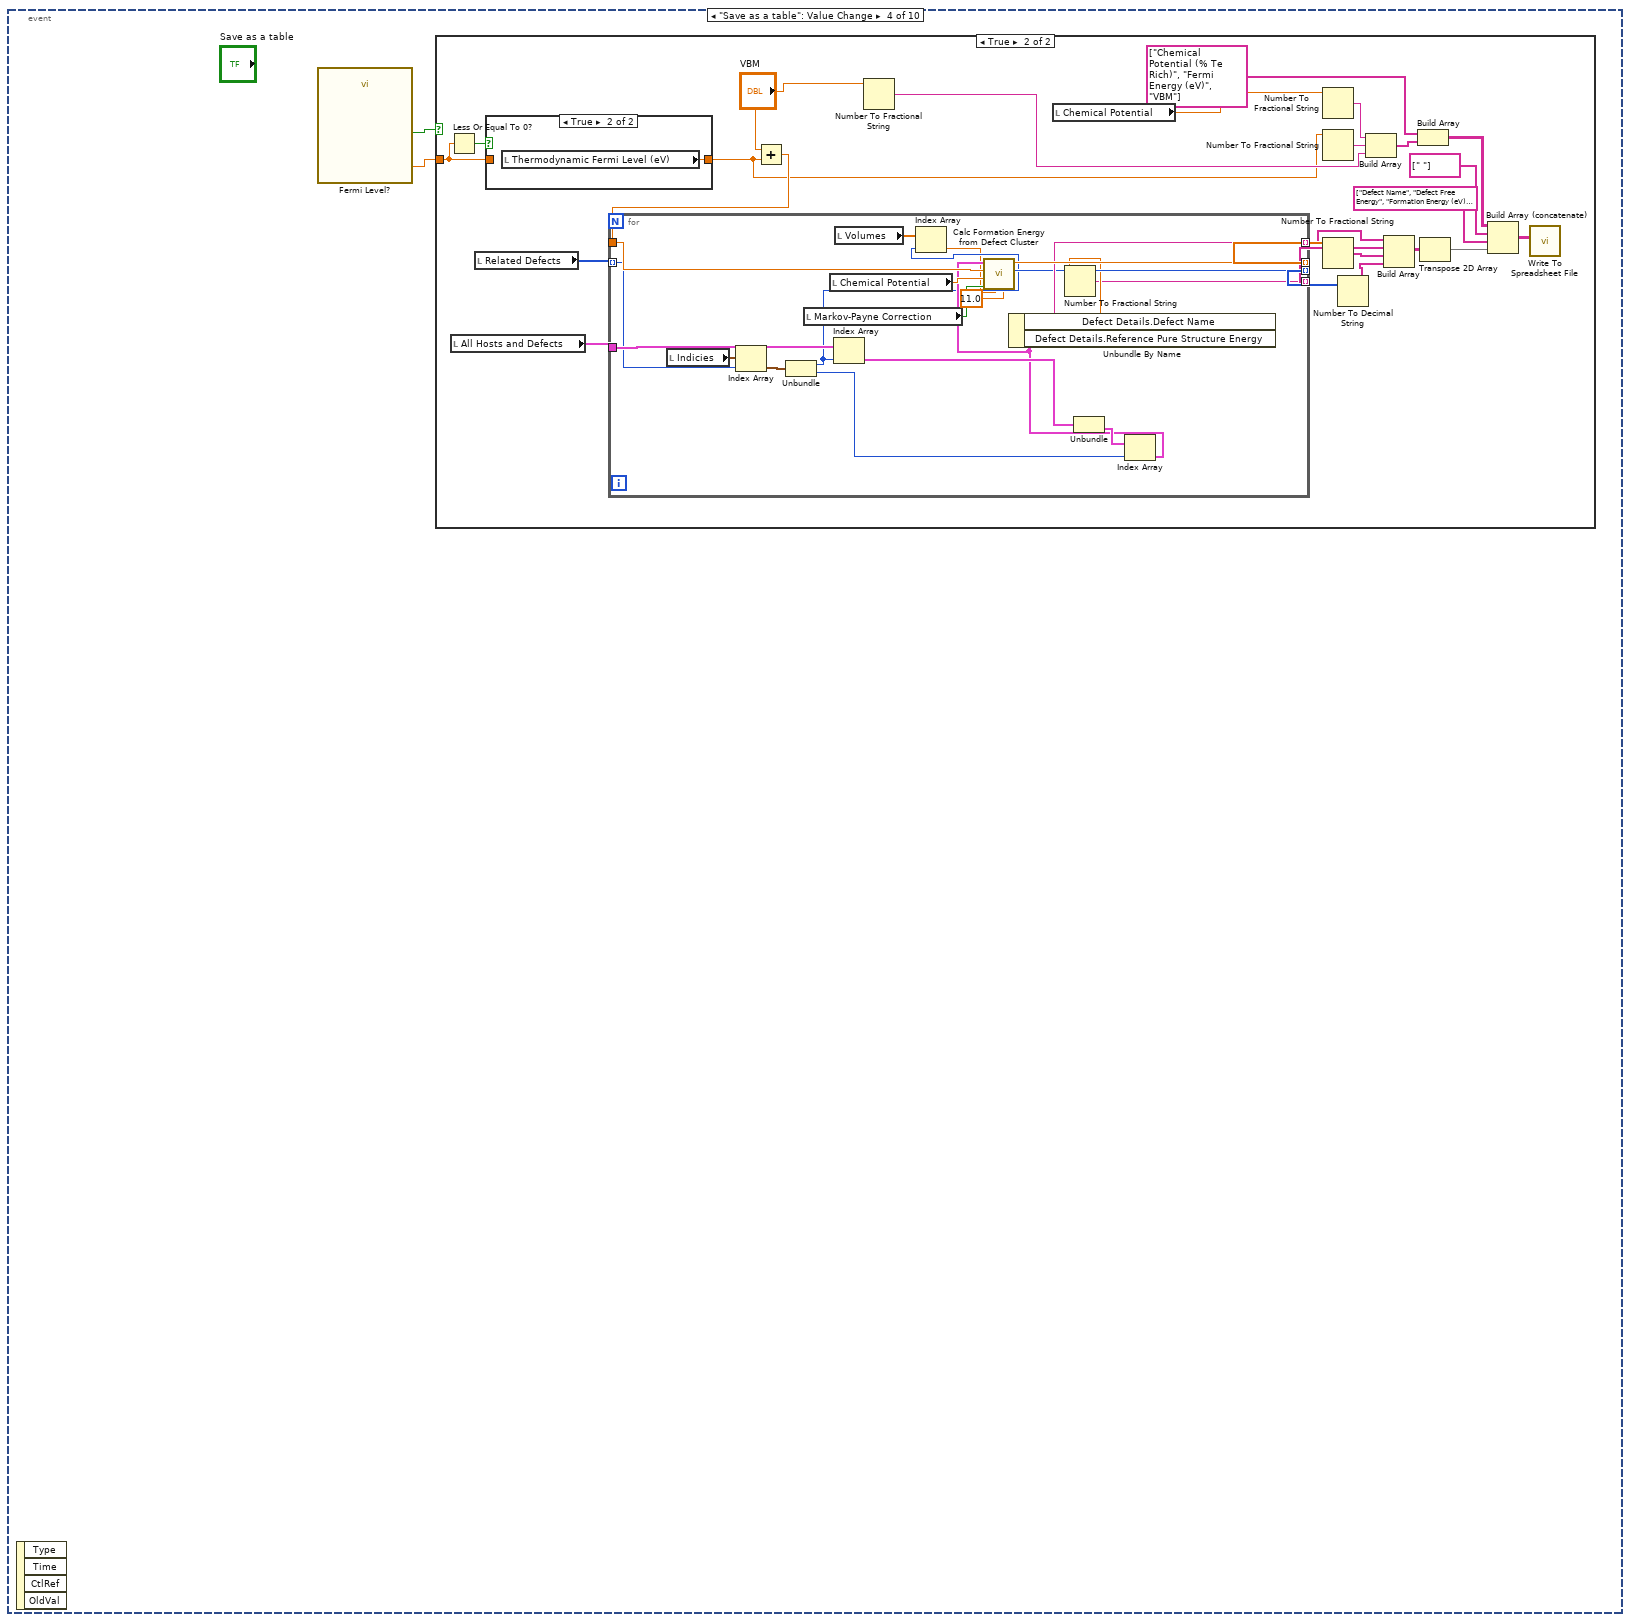
[diagram p14: hidden frame]
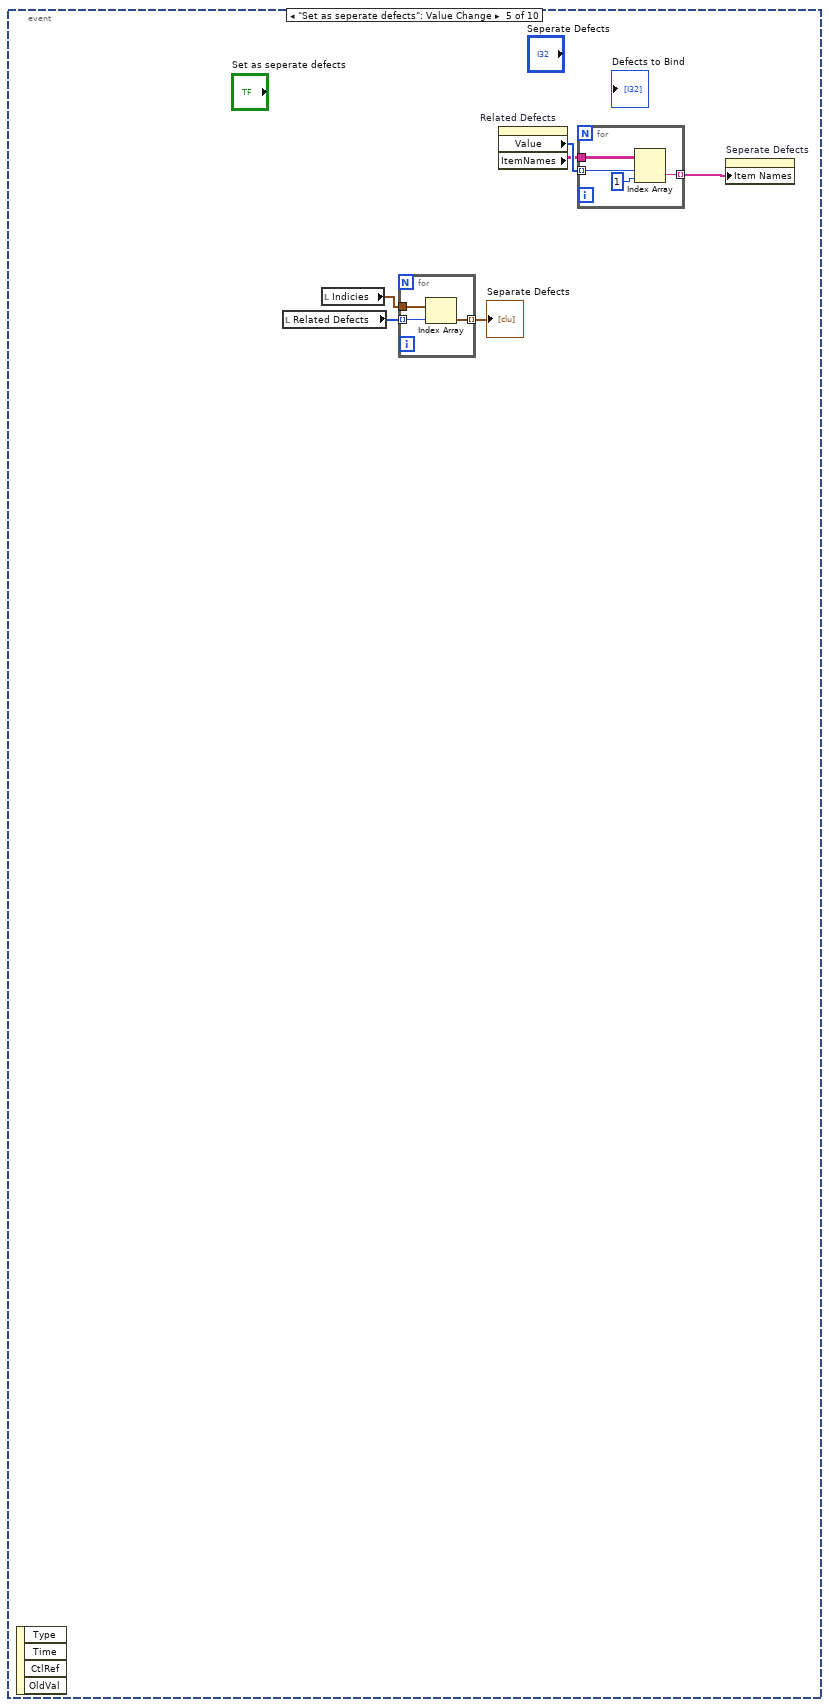
[diagram p17: hidden frame]
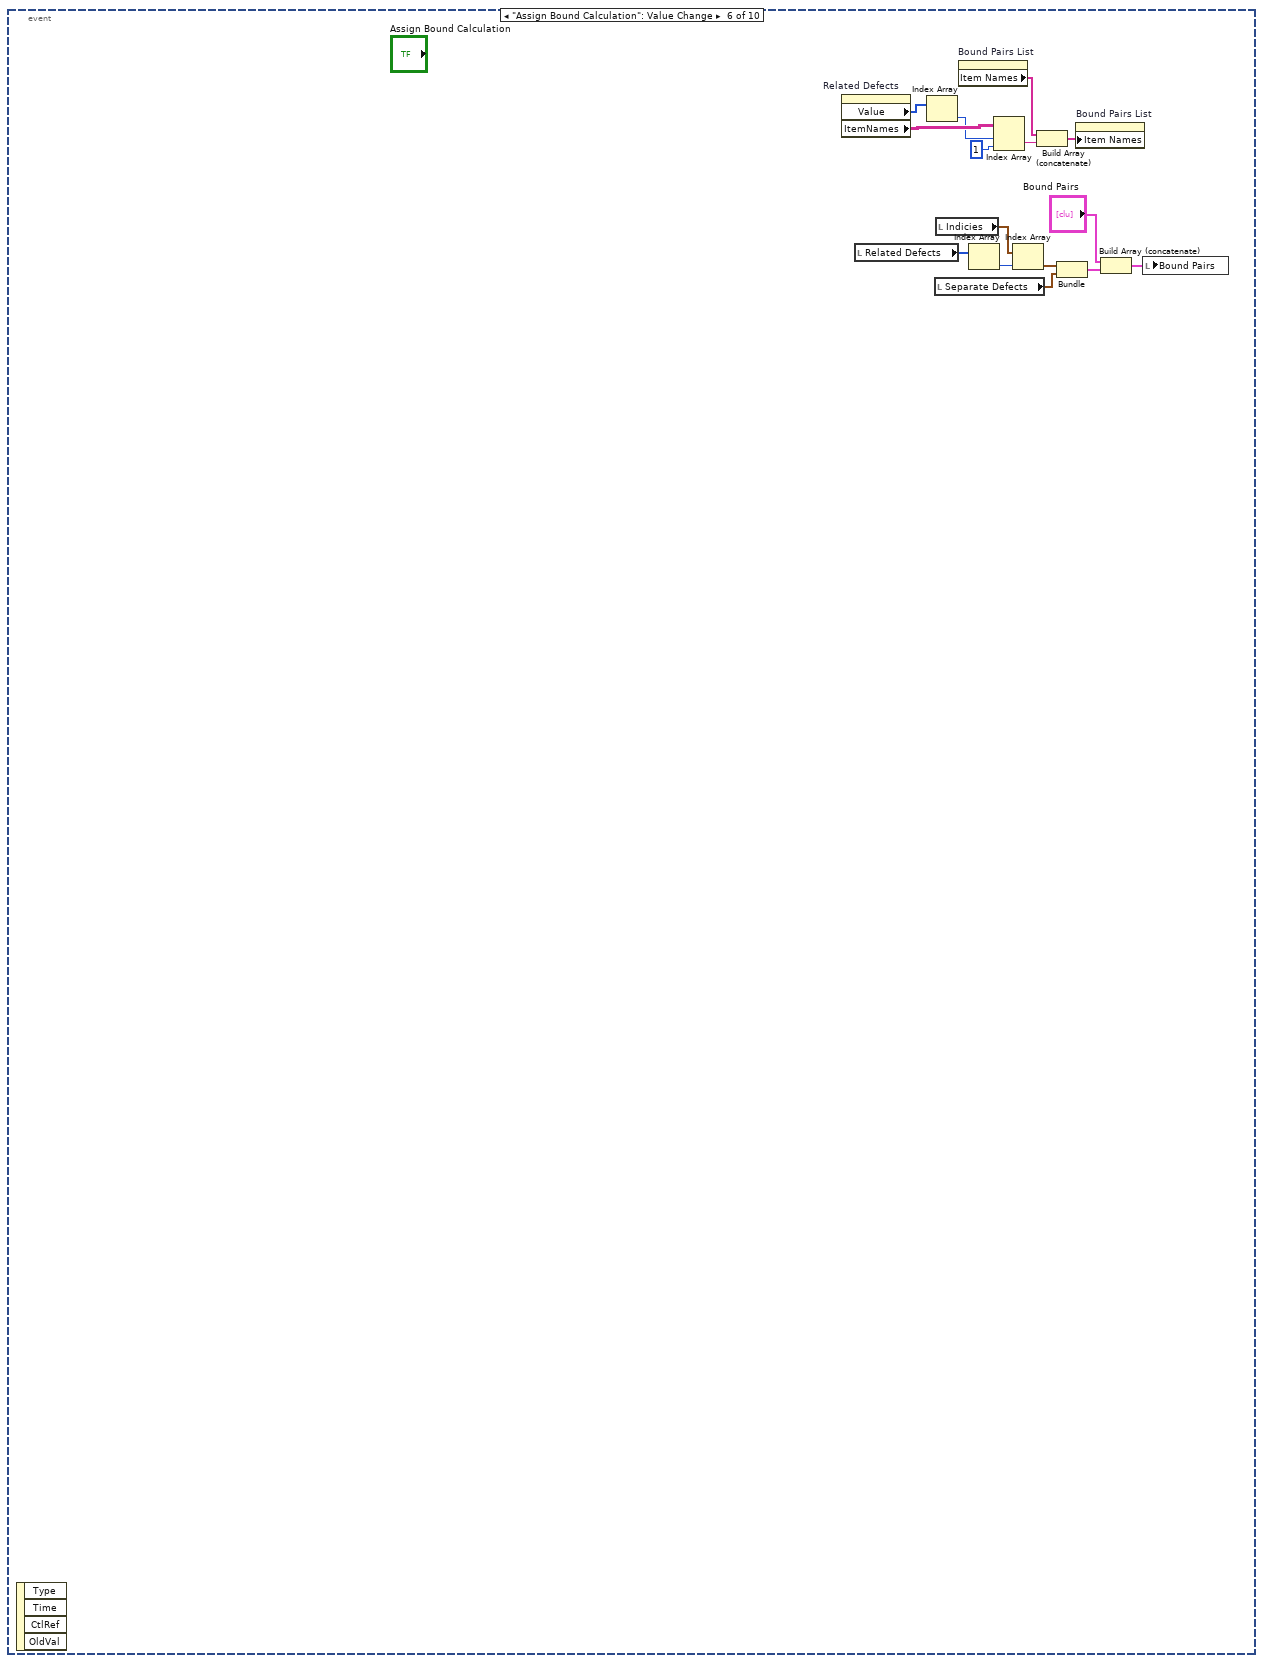
[diagram p18: hidden frame]
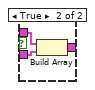
[diagram p19: hidden frame]
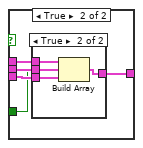
[diagram p20: hidden frame]
diagram:
  n1 = call-poly <vilib>:"DB Tools Open Connection.vi"("connection information"="UDL") -> ("error out"=w6:errorcluster, "connection reference"=w14:T6)  [unwired: 7 in]
  n2 = call-poly <vilib>:"DB Tools Execute Query.vi"("error in (no error)"=w6, "SQL query"="SELECT DISTINCT [0D_Point_Defects].Defect_Free_Structure_ID, [0D_Point_Defects].Defect_Free_Structure_Name, [0D_Point_Defects].[Defect_Free_Energy_(eV)]\nFROM [0D_Point_Defects];\n", "connection reference"=w14) -> ("error out"=w16:errorcluster, "recordset reference"=w13:T9)  [unwired: 5 in]
  n3 = call "Column Headers from SQL Query Recordset.vi"("error in (no error)"=w16, "recordset reference"=w13) -> ("error out"=w15:errorcluster, "columns"=w7:string[], "Recordset reference Out"=w12:T9)  [unwired: 6 in, 1 out]
  n4 = call-poly <vilib>:"DB Tools Fetch Recordset Data.vi"("error in (no error)"=w15, "recordset reference"=w12) -> ("error out"=w17:errorcluster, "recordset data"=w9:variant[][], "recordset reference out"=w11:T9)  [unwired: 3 in]
  n5 = for {
    tunnel: w9 -> [w20] mode=indexing
    tunnel: [w19] -> w8 mode=indexing
    n6 = for {
      tunnel: w20 -> [w23] mode=indexing
      tunnel: [w21] -> w19 mode=indexing
      n7 = xnode "Database Variant To Data"("database variant"=w23, "type"="") -> ("data"=w21:string)  [unwired: 1 in, 1 out]
    }
  }
  n8 = call-poly <vilib>:"DB Tools Free Object.vi"("error in (no error)"=w17, "recordset reference"=w11) -> ("connection reference"=w1:T6)  [unwired: 8 in, 1 out]
  "connection reference" <- w1
  n9 = call <vilib>:"Create Object.vi"("Name"="Base") -> ("error out"=w2:errorcluster, "Scene:New Object"=→"Base Object":refnum<vi>)  [unwired: 1 in, 8 out]
  n10 = property on="Pure Structures with defects" class="MCListbox (strict)"(error in=w2, "ColHdrString"=w7, "ItemNames"=w8) -> (error out=w5:errorcluster)  [unwired: 1 in, 1 out]
  n11 = while {
    tunnel: w5 -> [_]
    tunnel: w1 -> [_]
    stop <- FALSE stop-if-true
    n12 = event shown="[6] \"Bound Pairs List\": Value Change" {
      selector: _ -> [_ _ _ _ _ _ _ _ _ _]
      dyn-events: _ -> [_ _ _ _ _ _ _ _ _ _]
      timeout: 60000 -> [_ _ _ _ _ _ _ _ _ _]
      event Timeout {
        n13 = event-data() -> ()  [unwired: 1 in, 2 out]
        n14 = Wait (ms)(milliseconds to wait=u32 10) -> ()  [unwired: 1 out]
      }
      event "Pure Structures with defects", "Chemical Potential", "Chemical Potential 2", "Thermodynamic Fermi Level": Value Change {
        w61 = string[] [] ("Item Names")
        w77 = -1.0 ("Thermodynamic Fermi Level (eV)")
        w60 = string[][] []
        w82 = T11 {"Name"="Thermodynamic Fermi Level", "Color"=0, "Style"=2, "Point Style"=13, "Name Visible"=TRUE, "Allow Drag"=TRUE, "Cursor Mode"=0, "Plot"=0, "Index"=0, "Position"={"X"=2.4701149425287356, "Y"=0.0}, "X Scale"=0, "Y Scale"=0, "Watch Plots"=[], "Watch All Plots"=FALSE, "Plot Area"=0, "Label Offset"={"X"=0.016091954022988464, "Y"=2.3061224489795915}} ("element")
        n15 = event-data() -> ()  [unwired: 1 in, 3 out]
        n16 = property on="Pure Structures with defects" class="MCListbox (strict)"() -> ("ItemNames"=w91:string[][])  [unwired: 2 in, 2 out]
        n17 = local read "connection reference"() -> (w87:T6)
        n18 = Index Array(array=w91, index (col) #1=0 ("disabled index (col)")) -> (element #1=w88:string[], element #2=w71:string[])  [unwired: 3 in]
        n19 = for {
          tunnel: "Pure Structures with defects" -> [w97] mode=indexing
          tunnel: w88 -> [w129]
          shift-right: [w127] -> _
          shift-left: w87 -> [w128]
          shift-right: [w118] -> w66
          shift-left: w60 -> [w117]
          tunnel: "Calc Thermodynamic Fermi Level" -> [w116]
          shift-right: [w123] -> w76
          shift-left: w77 -> [w113]
          shift-right: [w124] -> w75
          shift-left: w77 -> [w112]
          tunnel: [w110] -> w74 mode=indexing
          shift-right: [w106] -> w72
          shift-left: cluster{i32, i32}[] [] -> [w105]
          tunnel: w71 -> [w104]
          tunnel: dbl[] [5230.5515143, 4360.60278, 2309.371815, 7792.576126] ("Volumes 2") -> [w99]
          tunnel: [w98] -> w63 mode=indexing
          shift-right: [w95] -> w59
          shift-left: w60 -> [w94]
          i -> [w108]
          n20 = Index Array(array=w129, index=w97) -> (element=w111:string)
          n21 = Index Array(array=w104, index=w97) -> (element=w103:string)
          n22 = Index Array(array=w99, index=w97) -> (element=w98:dbl)
          n23 = property on="Pure Structures with defects" class="MCListbox (strict)"() -> ("ItemNames"=w122:string[][])  [unwired: 2 in, 2 out]
          n24 = local read "Chemical Potential 2"() -> (w125:dbl)
          n25 = local read "Chemical Potential"() -> (w126:dbl)
          n26 = Equal?(x="Thermodynamic Fermi Level", y=w97) -> (x = y?=w115:bool)
          n27 = call "DB Get Defects from pure ID.vi"("Ignore Incomplete"="Ignore Incomplete", "Ignore Location"="Ignore Location", "Defect Free Structure ID"=w111, "connection reference in"=w128) -> ("String Data"=w96:string[][], "Defects Array"=w109:T12, "connection reference out"=w127:T6)  [unwired: 4 in, 1 out]
          n28 = Index Array(array=w122, index (row)=w97, index (col)=1 ("disabled index (col)")) -> (element=w120:string)
          n29 = Index Array(array=w99, index="Thermodynamic Fermi Level") -> (element=w100:dbl)
          n30 = for {
            tunnel: [w143] -> w119 mode=indexing
            tunnel: w120 -> [w142]
            tunnel: w109 -> [w141] mode=indexing
            tunnel: w108 -> [w139]
            tunnel: [w138] -> w107 mode=indexing
            i -> [w140]
            n31 = Unbundle By Name(w141) -> ("Defect Details"=w146:T13, "Charges and Energies"=w148:T14)
            n32 = Unbundle By Name(w146) -> ("Defect Name"=w145:string)
            n33 = for {
              tunnel: w148 -> [w154] mode=indexing
              shift-right: [w153] -> w144
              shift-left: "" -> [w152]
              n34 = Unbundle By Name(w154) -> ("Net Charge"=w151:i32)
              n35 = Number To Decimal String(number=w151) -> (decimal integer string=w150:string)  [unwired: 1 in]
              n36 = Concatenate Strings(w152, w150, ", " ("string")) -> (w153:string)
            }
            n37 = Build Array(w142, w145, w144) -> (w143:string[])
            n38 = Bundle(w139, w140) -> (w138:cluster{i32, i32})  [unwired: 1 in]
          }
          n39 = And(x=w116, y=w115) -> (x .and. y?=w114:bool)
          n40 = case shown="True" w114 {
            tunnel: w126 -> [_ w137]
            tunnel: w125 -> [_ w136]
            tunnel: [w130 w135] -> w124
            tunnel: [w131 w134] -> w123
            tunnel: w109 -> [_ w133]
            tunnel: w113 -> [w131 _]
            tunnel: w112 -> [w130 _]
            tunnel: w100 -> [_ w132]
            frame False {
            }
            frame True {
              n41 = call "Self-consistent charge neutrality.vi"("Volume (A³)"=w132, "Chemical Potential (0=Cd, 1=Te)"=w136, "Defects"=w133) -> ("Thermodynamic Fermi Level (eV) - VBM"=w134:dbl)  [unwired: 8 in]
              n42 = call "Self-consistent charge neutrality.vi"("Volume (A³)"=w132, "Chemical Potential (0=Cd, 1=Te)"=w137, "Defects"=w133) -> ("Thermodynamic Fermi Level (eV) - VBM"=w135:dbl)  [unwired: 8 in]
            }
          }
          n43 = Bundle(w103, "Defects Array"=w109) -> (w110:T15)  [unwired: 1 in]
          n44 = Build Array (concatenate)(w94, w96) -> (w95:string[][])
          n45 = Build Array (concatenate)(w117, w119) -> (w118:string[][])
          n46 = Build Array (concatenate)(w105, w107) -> (w106:cluster{i32, i32}[])
        }
        "Thermodynamic Fermi Level (eV)" <- w75
        "All Hosts and Defects" <- w74
        "Indicies" <- w72
        "Array" <- w66
        "Table Control" <- w59
        n47 = property on="Bound Pairs List" class="LstBox (strict)"("Item Names"=w61) -> ()  [unwired: 2 in, 2 out]
        n48 = property on="Seperate Defects" class="LstBox (strict)"("Item Names"=w61) -> ()  [unwired: 2 in, 2 out]
        n49 = local write "Bound Pairs"(T1 [] ("Bound Pairs")) -> ()
        n50 = Array To Spreadsheet String(delimiter (Tab)=",", array=w66, 3:"\\s" ("format string")) -> (spreadsheet string=→"spreadsheet string":string)
        n51 = disable-structure shown="Enabled" {
          disable-tunnel: [_ w92] -> w81
          frame Disabled {
          }
          frame Enabled {
            n52 = local read "Related Defects"() -> (w92:i32[])
          }
        }
        n53 = Index Array(array=w66, index (col)=1 ("disabled index (col)")) -> (element=w70:string[])  [unwired: 1 in]
        n54 = property on="Related Defects" class="MCListbox (strict)"("ColHdrString"=string[] ["Defect Free Structure", "Defect Name", "Net Charges"] ("Column Header Strings[]"), "ItemNames"=w66) -> (error out=w79:errorcluster)  [unwired: 2 in, 1 out]
        n55 = local write "Volumes"(w63) -> ()
        n56 = Bundle By Name(cluster=w82, "Position.X"=w76) -> (w83:T11)
        n57 = Bundle By Name(cluster=w82, "Position.X"=w75) -> (w85:T11)
        n58 = property on="Related Defects" class="MCListbox (strict)"(error in=w79, "Val(Sgnl)"=w81) -> ()  [unwired: 1 in, 2 out]
        n59 = Build Array(w83) -> (w84:T16)
        n60 = Build Array(w85) -> (w86:T16)
        n61 = property on="Defect" class="CmbBox"("Strings[]"=w70) -> ()  [unwired: 2 in, 2 out]
        n62 = property on="Te Rich Limit" class="XYGraph (strict)"("CrsrList"=w84) -> ()  [unwired: 2 in, 2 out]
        n63 = property on="Cd Rich Limit" class="XYGraph (strict)"("CrsrList"=w86) -> ()  [unwired: 2 in, 2 out]
      }
      event "Related Defects", "Show Charge Transitions", "Markov-Payne Correction": Value Change {
        w172 = T17 []
        n64 = event-data() -> ()  [unwired: 1 in, 4 out]
        n65 = local read "All Hosts and Defects"() -> (w162:T4)
        n66 = for {
          N -> [w214]
          tunnel: w162 -> [w200]
          tunnel: [w219] -> w167 mode=indexing
          tunnel: [w217] -> w169 mode=indexing
          tunnel: [w184] -> w159 mode=indexing
          tunnel: [w214] -> w176
          tunnel: "Related Defects" -> [w202] mode=indexing
          shift-right: [w208] -> w171
          shift-left: w172 -> [w212]
          tunnel: T10 {"Name"="0 / +1", "Color"=0, "Style"=4, "Point Style"=1, "Name Visible"=TRUE, "Allow Drag"=TRUE, "Annotation Mode"=0, "Plot"=-1, "Index"=0, "Position"={"X"=2.0, "Y"=1.0}, "X Scale"=0, "Y Scale"=0, "Show Arrow"=FALSE, "Lock Name"=FALSE, "Plot Area"=0, "Label Offset"={"X"=0.0, "Y"=0.05}} ("element 2") -> [w211]
          shift-right: [w207] -> w170
          shift-left: w172 -> [w209]
          tunnel: [w204] -> w164 mode=indexing
          shift-right: [w193] -> w160
          shift-left: string[][] [] -> [w192]
          tunnel: [w183] -> w155 mode=indexing
          n67 = local read "Indicies"() -> (w203:cluster{i32, i32}[])
          n68 = local read "VBM"() -> (w188:dbl)
          n69 = Add(x=w188, y=1.5) -> (x+y=w187:dbl)
          n70 = Index Array(array=w203, index=w202) -> (element=w201:cluster{i32, i32})
          n71 = call "Start and End to Array 2.vi"("Sweep Style"=enum16{"Linear Step", "Linear Pts", "Log Pts"}."Linear Pts", "Step or # Pts"=100.0, "End"=w187, "Start"=w188) -> ("Array"=w210:dbl[])  [unwired: 7 in]
          n72 = Unbundle(w201) -> (w191:i32, w197:i32)
          n73 = Index Array(array="Volumes", index=w191) -> (element=w189:dbl)
          n74 = Index Array(array=w200, index=w191) -> (element=w199:T18)
          n75 = Build Array (concatenate)(w210) -> (w206:dbl[])
          n76 = Unbundle(w199) -> ("Defect Free Name"=w185:string, "Defects Array"=w198:T12)
          n77 = Index Array(array=w198, index=w197) -> (element=w196:T19)
          n78 = Unbundle By Name(w196) -> ("Defect Details.Defect Name"=w184:string, "Charges and Energies"=w195:T14)
          n79 = case shown="True" "Show Charge Transitions" {
            tunnel: w196 -> [_ w242]
            tunnel: w212 -> [_ w240]
            tunnel: w211 -> [_ w241]
            tunnel: w209 -> [_ w237]
            tunnel: [_ w238] -> w208
            tunnel: [_ w235] -> w207
            tunnel: w184 -> [_ w233]
            tunnel: [_ w232] -> w204
            tunnel: w189 -> [_ w231]
            frame False {
            }
            frame True {
              n80 = local read "Markov-Payne Correction"() -> (w230:bool)
              n81 = local read "VBM"() -> (w229:dbl)
              n82 = call "Find Charge Transitions.vi"("Dielectric Constant"=11.0, "Volume (A³)"=w231, "Markov-Payne Corrections"=w230, "VBM"=w229, "Defect Data"=w242) -> ("Transitions"=w234:T20)  [unwired: 6 in]
              n83 = Bundle("Defect Name"=w233, "Transitions"=w234) -> (w232:T21)  [unwired: 1 in]
              n84 = for {
                tunnel: w234 -> [w257] mode=indexing
                tunnel: w241 -> [w255]
                tunnel: [w251] -> w239 mode=indexing
                tunnel: [w250] -> w236 mode=indexing
                n85 = local read "Chemical Potential 2"() -> (w244:dbl)
                n86 = local read "Chemical Potential"() -> (w247:dbl)
                n87 = Unbundle(w257) -> ("Transition"=w254:string, "Fermi Energy (eV)"=w253:dbl, "Formation Energy, Cd Rich (eV)"=w249:dbl, "Formation Energy, Te Rich (eV)"=w248:dbl)
                n88 = Build Array(w249, w248) -> (w245:dbl[])
                n89 = Interpolate 1D Array(1:w247, 2:w245) -> (0:w246:dbl)
                n90 = Interpolate 1D Array(1:w244, 2:w245) -> (0:w243:dbl)
                n91 = Bundle("Fermi Energy (eV)"=w253, w246) -> (w256:cluster{"Fermi Energy (eV)":dbl, dbl})  [unwired: 1 in]
                n92 = Bundle("Fermi Energy (eV)"=w253, w243) -> (w252:cluster{"Fermi Energy (eV)":dbl, dbl})  [unwired: 1 in]
                n93 = Bundle By Name(cluster=w255, "Name"=w254, "Position"=w256) -> (w251:T10)
                n94 = Bundle By Name(cluster=w255, "Name"=w254, "Position"=w252) -> (w250:T10)
              }
              n95 = Build Array (concatenate)(w240, w239) -> (w238:T17)
              n96 = Build Array (concatenate)(w237, w236) -> (w235:T17)
            }
          }
          n97 = for {
            tunnel: w206 -> [w264] mode=indexing
            tunnel: [w263] -> w220 mode=indexing
            tunnel: [w262] -> w218 mode=indexing
            tunnel: w196 -> [w261]
            tunnel: w189 -> [w259]
            w258 = 11.0 ("Dielectric Constant")
            n98 = call "Calc Formation Energy from Defect Cluster.vi"("Dielectric Constant"=w258, "Volume (A³)"=w259, "Markov-Payne Correction"="Markov-Payne Correction", "Chemical Potential"="Chemical Potential", "Fermi Level (eV)"=w264, "Defect Data"=w261) -> ("Formation Energy (eV)"=w263:dbl)  [unwired: 4 in, 1 out]
            n99 = call "Calc Formation Energy from Defect Cluster.vi"("Dielectric Constant"=w258, "Volume (A³)"=w259, "Markov-Payne Correction"="Markov-Payne Correction", "Chemical Potential"="Chemical Potential 2", "Fermi Level (eV)"=w264, "Defect Data"=w261) -> ("Formation Energy (eV)"=w262:dbl)  [unwired: 4 in, 1 out]
          }
          n100 = for {
            tunnel: w195 -> [w227] mode=indexing
            tunnel: w185 -> [w224]
            tunnel: w184 -> [w223]
            tunnel: [w222] -> w194 mode=indexing
            n101 = Unbundle By Name(w227) -> ("Net Charge"=w226:i32, "Structure ID"=w221:string)
            n102 = Number To Decimal String(number=w226) -> (decimal integer string=w225:string)  [unwired: 1 in]
            n103 = Build Array(w224, w223, w225, w221) -> (w222:string[])
          }
          n104 = Build Array(w185, w184) -> (w183:string[])
          n105 = Build Array (concatenate)(w192, w194) -> (w193:string[][])
          n106 = Subtract(x=w206, y=w188) -> (x-y=w205:dbl[])
          n107 = Bundle(w205, w218) -> (w217:cluster{dbl[], dbl[]})  [unwired: 1 in]
          n108 = Bundle(w205, w220) -> (w219:cluster{dbl[], dbl[]})  [unwired: 1 in]
        }
        "Cd Rich Limit" <- w167
        "Te Rich Limit" <- w169
        "Array 2" <- w164
        "Plot Names" <- w155
        n109 = local read "Plots Tab"() -> (w168:T7)
        n110 = case shown="\"Binding Energy\"" w168 {
          frame "Formation Energies vs Fermi", Default {
          }
          frame "Binding Energy" {
            n111 = property on="Plot Binding Energy" class="Bool (strict)"("Val(Sgnl)"=TRUE ("Value (Signaling)")) -> ()  [unwired: 2 in, 2 out]
          }
          frame "Charge Transition Levels" {
          }
          frame "Atomic Structure" {
          }
        }
        n112 = property on="Atomic Structures" class="MCListbox (strict)"("ItemNames"=w160) -> ()  [unwired: 2 in, 2 out]
        n113 = property on="Te Rich Limit" class="XYGraph (strict)"("AnntList"=w170) -> ()  [unwired: 2 in, 2 out]
        n114 = property on="Cd Rich Limit" class="XYGraph (strict)"("AnntList"=w171) -> ()  [unwired: 2 in, 2 out]
        n115 = control-ref of="Defect Energy Levels"() -> (w165:refnum<vi>)
        n116 = disable-structure shown="Enabled" {
          disable-tunnel: w164 -> [w178 w181]
          disable-tunnel: [w177 w181] -> w163
          frame Disabled {
            n117 = Decimate 1D Array(w178) -> (w180:T2, w179:T2)
            n118 = Build Array (concatenate)(w180, w179) -> (w177:T2)
          }
          frame Enabled {
          }
        }
        n119 = call "Num of Colors to Color Array.vi"("# of Colors"=w176, "Color Array Type"="Color Array Type") -> ("Colors Array"=w157:u32[])  [unwired: 3 in]
        n120 = call "Make Defect Energy Transition Plot.vi"("Buckets"="Buckets", "All Defects and Transitions"=w163, "XY Graph Reference"=w165) -> ()  [unwired: 9 in]
        n121 = control-ref of="Te Rich Limit"() -> (w166:refnum<vi>)
        n122 = control-ref of="Cd Rich Limit"() -> (w175:refnum<vi>)
        n123 = call "Format XY Plot.vi"("Colors Array"=w157, "Plot Names"=w159, "XY Graph Reference"=w166) -> ()  [unwired: 9 in]
        n124 = call "Format XY Plot.vi"("Colors Array"=w157, "Plot Names"=w159, "XY Graph Reference"=w175) -> ()  [unwired: 9 in]
      }
      event "Save as a table": Value Change {
        n125 = event-data() -> ()  [unwired: 1 in, 4 out]
        n126 = call "Fermi Level?"() -> ("Fermi Level"=w267:dbl, "OK"=w268:bool)  [unwired: 17 in, 1 out]
        n127 = case shown="True" w268 {
          tunnel: w267 -> [_ w276]
          frame False {
          }
          frame True {
            n128 = Less Or Equal To 0?(x=w276) -> (x <= 0?=w277:bool)
            n129 = local read "All Hosts and Defects"() -> (w269:T4)
            n130 = local read "Related Defects"() -> (w293:i32[])
            n131 = case shown="True" w277 {
              tunnel: [w294 w295] -> w270
              tunnel: w276 -> [w294 _]
              frame False {
              }
              frame True {
                n132 = local read "Thermodynamic Fermi Level (eV)"() -> (w295:dbl)
              }
            }
            n133 = Add(x="VBM", y=w270) -> (x+y=w282:dbl)
            n134 = for {
              tunnel: w293 -> [w303] mode=indexing
              tunnel: [w314] -> w292 mode=indexing
              tunnel: [w313] -> w291 mode=indexing
              tunnel: w282 -> [w312]
              tunnel: [w311] -> w275 mode=indexing
              tunnel: [w309] -> w273 mode=indexing
              tunnel: w269 -> [w304]
              n135 = local read "Indicies"() -> (w308:cluster{i32, i32}[])
              n136 = Index Array(array=w308, index=w303) -> (element=w307:cluster{i32, i32})
              n137 = Unbundle(w307) -> (w298:i32, w305:i32)
              n138 = local read "Markov-Payne Correction"() -> (w300:bool)
              n139 = local read "Chemical Potential"() -> (w315:dbl)
              n140 = Index Array(array=w304, index=w298) -> (element=w306:T18)
              n141 = local read "Volumes"() -> (w299:dbl[])
              n142 = Index Array(array=w299, index=w298) -> (element=w297:dbl)
              n143 = Unbundle(w306) -> ("Defects Array"=w302:T12)  [unwired: 1 out]
              n144 = Index Array(array=w302, index=w305) -> (element=w301:T19)
              n145 = call "Calc Formation Energy from Defect Cluster.vi"("Dielectric Constant"=11.0, "Volume (A³)"=w297, "Markov-Payne Correction"=w300, "Chemical Potential"=w315, "Fermi Level (eV)"=w312, "Defect Data"=w301) -> ("Net Charge"=w311:i32, "Formation Energy (eV)"=w314:dbl)  [unwired: 4 in]
              n146 = Unbundle By Name(w301) -> ("Defect Details.Defect Name"=w313:string, "Defect Details.Reference Pure Structure Energy"=w310:dbl)
              n147 = Number To Fractional String(number=w310) -> (F-format string=w309:string)  [unwired: 3 in]
            }
            n148 = Number To Fractional String(number="VBM") -> (F-format string=w271:string)  [unwired: 3 in]
            n149 = local read "Chemical Potential"() -> (w287:dbl)
            n150 = Number To Fractional String(number=w287) -> (F-format string=w286:string)  [unwired: 3 in]
            n151 = Number To Fractional String(number=w270) -> (F-format string=w288:string)  [unwired: 3 in]
            n152 = Number To Fractional String(number=w292) -> (F-format string=w290:string[])  [unwired: 3 in]
            n153 = Number To Decimal String(number=w275) -> (decimal integer string=w274:string[])  [unwired: 1 in]
            n154 = Build Array(w286, w288, w271) -> (w284:string[])
            n155 = Build Array(w291, w273, w290, w274) -> (w289:string[][])
            n156 = Build Array(string[] ["Chemical Potential (% Te Rich)", "Fermi Energy (eV)", "VBM"], w284) -> (w283:string[][])
            n157 = Transpose 2D Array(2D array=w289) -> (transposed array=w279:string[][])
            n158 = Build Array (concatenate)(w283, string[] [" "] ("element"), string[] ["Defect Name", "Defect Free Energy", "Formation Energy (eV)", "Net Charge"], w279) -> (w281:string[][])
            n159 = call-poly <vilib>:"Write To Spreadsheet File.vi"("2D data"=w281) -> ()  [unwired: 7 in, 1 out]
          }
        }
      }
      event "Set as seperate defects": Value Change {
        n160 = event-data() -> ()  [unwired: 1 in, 4 out]
        n161 = local read "Related Defects"() -> (w318:i32[])
        n162 = local read "Indicies"() -> (w317:cluster{i32, i32}[])
        n163 = for {
          tunnel: w318 -> [w323] mode=indexing
          tunnel: w317 -> [w324]
          tunnel: [w322] -> w316 mode=indexing
          n164 = Index Array(array=w324, index=w323) -> (element=w322:cluster{i32, i32})
        }
        "Separate Defects" <- w316
        n165 = property on="Related Defects" class="MCListbox (strict)"() -> ("Value"=w321:i32[], "ItemNames"=w320:string[][])  [unwired: 2 in, 2 out]
        n166 = for {
          tunnel: w321 -> [w328] mode=indexing
          tunnel: w320 -> [w327]
          tunnel: [w325] -> w319 mode=indexing
          n167 = Index Array(array=w327, index (row)=w328, index (col)=1 ("disabled index (col)")) -> (element=w325:string)
        }
        n168 = property on="Seperate Defects" class="LstBox (strict)"("Item Names"=w319) -> ()  [unwired: 2 in, 2 out]
      }
      event "Assign Bound Calculation": Value Change {
        n169 = event-data() -> ()  [unwired: 1 in, 4 out]
        n170 = property on="Related Defects" class="MCListbox (strict)"() -> ("Value"=w333:i32[], "ItemNames"=w335:string[][])  [unwired: 2 in, 2 out]
        n171 = local read "Related Defects"() -> (w343:i32[])
        n172 = Index Array(array=w333) -> (element=w332:i32)  [unwired: 1 in]
        n173 = local read "Separate Defects"() -> (w339:cluster{i32, i32}[])
        n174 = local read "Indicies"() -> (w342:cluster{i32, i32}[])
        n175 = property on="Bound Pairs List" class="LstBox (strict)"() -> ("Item Names"=w331:string[])  [unwired: 2 in, 2 out]
        n176 = Index Array(array=w343) -> (element=w341:i32)  [unwired: 1 in]
        n177 = Index Array(array=w335, index (row)=w332, index (col)=1 ("disabled index (col)")) -> (element=w329:string)
        n178 = Index Array(array=w342, index=w341) -> (element=w340:cluster{i32, i32})
        n179 = Build Array (concatenate)(w331, w329) -> (w330:string[])
        n180 = Bundle(w340, "Separate Defects"=w339) -> (w337:T22)  [unwired: 1 in]
        n181 = property on="Bound Pairs List" class="LstBox (strict)"("Item Names"=w330) -> ()  [unwired: 2 in, 2 out]
        n182 = Build Array (concatenate)("Bound Pairs", w337) -> (w336:T1)
        n183 = local write "Bound Pairs"(w336) -> ()
      }
      event "Bound Pairs List": Value Change {
        n184 = event-data() -> ()  [unwired: 1 in, 4 out]
        n185 = local read "VBM"() -> (w345:dbl)
        n186 = Add(x=w345, y=1.5) -> (x+y=w344:dbl)
        n187 = local read "All Hosts and Defects"() -> (w362:T4)
        n188 = call "Start and End to Array 2.vi"("Sweep Style"=enum16{"Linear Step", "Linear Pts", "Log Pts"}."Linear Pts", "Step or # Pts"=30.0, "End"=w344, "Start"=w345) -> ("Array"=w364:dbl[])  [unwired: 7 in]
        n189 = local read "Markov-Payne Correction"() -> (w361:bool)
        n190 = local read "Bound Pairs"() -> (w366:T1)
        n191 = Subtract(x=w364, y=w345) -> (x-y=w363:dbl[])
        n192 = for {
          tunnel: "Bound Pairs List" -> [w406] mode=indexing
          tunnel: w366 -> [w407]
          tunnel: w364 -> [w395]
          tunnel: "Binding Energy Chem Pot" -> [w394]
          tunnel: w363 -> [w386]
          tunnel: w362 -> [w396]
          tunnel: w361 -> [w393]
          shift-right: [w374] -> w360
          shift-left: cluster{dbl[], dbl[]}[] [] -> [w375]
          shift-right: [w379] -> w357
          shift-left: string[] [] -> [w378]
          n193 = Index Array(array=w407, index=w406) -> (element=w405:T23)
          n194 = Unbundle(w405) -> ("Bound Pair"=w397:T24, "Separate Defects"=w404:T25)
          n195 = local read "Volumes"() -> (w401:dbl[])
          n196 = for {
            tunnel: w404 -> [w438]
            tunnel: w395 -> [w437] mode=indexing
            tunnel: w394 -> [w436]
            tunnel: w396 -> [w439]
            tunnel: w393 -> [w435]
            tunnel: [w433] -> w388 mode=indexing
            n197 = for {
              tunnel: w439 -> [w453]
              tunnel: w438 -> [w452] mode=indexing
              tunnel: w437 -> [w447]
              tunnel: w436 -> [w446]
              tunnel: w435 -> [w445]
              tunnel: [w440] -> w434 mode=indexing
              n198 = Unbundle(w452) -> ("Host Crystal Index"=w443:i32, "Defect Index"=w449:i32)
              n199 = local read "Volumes"() -> (w444:dbl[])
              n200 = Index Array(array=w453, index=w443) -> (element=w451:T18)
              n201 = Index Array(array=w444, index=w443) -> (element=w442:dbl)
              n202 = Unbundle(w451) -> ("Defects Array"=w450:T12)  [unwired: 1 out]
              n203 = Index Array(array=w450, index=w449) -> (element=w448:T19)
              n204 = call "Calc Formation Energy from Defect Cluster.vi"("Dielectric Constant"=11.0, "Volume (A³)"=w442, "Markov-Payne Correction"=w445, "Chemical Potential"=w446, "Fermi Level (eV)"=w447, "Defect Data"=w448) -> ("Formation Energy (eV)"=w440:dbl)  [unwired: 4 in, 1 out]
            }
            n205 = Add Array Elements(numeric array=w434) -> (sum=w433:dbl)
          }
          n206 = Unbundle(w397) -> ("Host Crystal Index"=w402:i32, "Defect Index"=w400:i32)
          n207 = Index Array(array=w396, index=w402) -> (element=w398:T18)
          n208 = Index Array(array=w401, index=w402) -> (element=w403:dbl)
          n209 = Unbundle(w398) -> ("Defects Array"=w399:T12)  [unwired: 1 out]
          n210 = Index Array(array=w399, index=w400) -> (element=w385:T19)
          n211 = for {
            tunnel: w385 -> [w432]
            tunnel: w395 -> [w431] mode=indexing
            tunnel: w394 -> [w430]
            tunnel: w393 -> [w429]
            tunnel: [w428] -> w389 mode=indexing
            tunnel: w403 -> [w426]
            n212 = call "Calc Formation Energy from Defect Cluster.vi"("Dielectric Constant"=11.0, "Volume (A³)"=w426, "Markov-Payne Correction"=w429, "Chemical Potential"=w430, "Fermi Level (eV)"=w431, "Defect Data"=w432) -> ("Formation Energy (eV)"=w428:dbl)  [unwired: 4 in, 1 out]
          }
          n213 = Bundle(w386, w389) -> (w392:cluster{dbl[], dbl[]})  [unwired: 1 in]
          n214 = Unbundle By Name(w385) -> ("Defect Details.Defect Name"=w382:string)
          n215 = Subtract(x=w388, y=w389) -> (x-y=w387:dbl[])
          n216 = Bundle(w386, w388) -> (w391:cluster{dbl[], dbl[]})  [unwired: 1 in]
          n217 = Bundle(w386, w387) -> (w390:cluster{dbl[], dbl[]})  [unwired: 1 in]
          n218 = Concatenate Strings("Binding of " ("string"), w382) -> (w380:string)
          n219 = Concatenate Strings("Separated " ("string"), w382) -> (w381:string)
          n220 = Build Array (concatenate)(w378, w382, w381, w380) -> (w379:string[])
          n221 = case shown="False" "Binding Energy" {
            tunnel: w392 -> [w410 w419]
            tunnel: w391 -> [w409 w418]
            tunnel: w390 -> [_ w417]
            tunnel: [w408 w416] -> w373
            tunnel: "Formation Energy" -> [w411 w415]
            frame False {
              n222 = case shown="False" w411 {
                tunnel: w410 -> [_ w414]
                tunnel: w409 -> [_ w413]
                tunnel: [_ w412] -> w408
                frame False {
                }
                frame True {
                  n223 = Build Array(w414, w413) -> (w412:cluster{dbl[], dbl[]}[])
                }
              }
            }
            frame True {
              n224 = case shown="True" w415 {
                tunnel: w419 -> [_ w425]
                tunnel: w418 -> [_ w424]
                tunnel: w417 -> [w421 w423]
                tunnel: [w420 w422] -> w416
                frame False {
                  n225 = Build Array(w421) -> (w420:cluster{dbl[], dbl[]}[])
                }
                frame True {
                  n226 = Build Array(w425, w424, w423) -> (w422:cluster{dbl[], dbl[]}[])
                }
              }
            }
          }
          n227 = Build Array (concatenate)(w375, w373) -> (w374:cluster{dbl[], dbl[]}[])
        }
        "Binding Energy" <- w360
        n228 = Array Size(array="Bound Pairs List") -> (size(s)=w349:i32)
        n229 = local read "Color Array Type"() -> (w370:T5)
        n230 = call "Num of Colors to Color Array.vi"("# of Colors"=w349, "Color Array Type"=w370) -> ("Colors Array"=w355:u32[])  [unwired: 3 in]
        n231 = Initialize Array(0, w349) -> (w352:i32[])
        n232 = Initialize Array(1, w349) -> (w351:i32[])
        n233 = Initialize Array(2, w349) -> (w348:i32[])
        n234 = Interleave 1D Arrays(w355, w355, w355) -> (w354:u32[])
        n235 = Interleave 1D Arrays(w352, w352, w351) -> (w353:i32[])
        n236 = control-ref of="Binding Energy"() -> (w369:refnum<vi>)
        n237 = Interleave 1D Arrays(w352, w351, w348) -> (w347:i32[])
        n238 = call "Format XY Plot.vi"("Active Y Scale (Left or Right)"=w353, "Line Styles"=w347, "Colors Array"=w354, "Plot Names"=w357, "XY Graph Reference"=w369) -> ()  [unwired: 7 in]
      }
      event "Atomic Structures", "Plot Atomic Structure", "Scale", "Atom Size", "Load in VESTA": Value Change {
        n239 = event-data() -> ()  [unwired: 1 in, 4 out]
        n240 = Less Than 0?(x="Atomic Structures") -> (x < 0?=w454:bool)
        n241 = case shown="False" w454 {
          tunnel: "Atomic Structures" -> [w458 _]
          frame False {
            n242 = local read "Base Object"() -> (w464:refnum<vi>)
            n243 = local read "connection reference"() -> (w459:T6)
            n244 = property on="Atomic Structures" class="MCListbox (strict)"() -> ("ItemNames"=w462:string[][])  [unwired: 2 in, 2 out]
            n245 = Close Reference(reference=w464) -> (error out=w463:errorcluster)  [unwired: 1 in]
            n246 = Index Array(array=w462, index (row)=w458, index (col)=3 ("disabled index (col)")) -> (element=w460:string)
            n247 = call <vilib>:"Create Object.vi"("error in (no error)"=w463, "Name"="Base") -> ("Scene:New Object"=w465:refnum<vi>)  [unwired: 9 out]
            n248 = call "Import Structure from DB.vi"("Structure ID"=w460, "connection reference"=w459) -> ("Loaded Structure"=w457:T3)  [unwired: 7 in, 2 out]
            "Loaded Structure" <- w457
            n249 = case shown="False" "Load in VESTA" {
              tunnel: w465 -> [w470 _]
              tunnel: w457 -> [w468 w473]
              frame False {
                n250 = call "Render Structure.vi"("Options"="Options", "Atom Size"="Atom Size", "Scale"="Scale", "Atomic Structure"=w468, "Base Object"=w470) -> ("Object with atoms"=w467:refnum<vi>)  [unwired: 6 in]
                "Atomic Structure" <- w467
                n251 = local write "Base Object"(w467) -> ()
              }
              frame True {
                n252 = call "Load Structure in VESTA.vi"("Atomic Structure"=w473) -> ()  [unwired: 11 in]
              }
            }
          }
          frame True {
          }
        }
      }
      event "Setup Camera": Value Change {
        n253 = event-data() -> ()  [unwired: 1 in, 4 out]
        n254 = local read "Loaded Structure"() -> (w489:T3)
        n255 = control-ref of="Atomic Structure"() -> (w474:refnum<vi>)
        n256 = Unbundle By Name(w489) -> ("Lattice vector a"=w479:dbl[], "Lattice vector b"=w478:dbl[], "Lattice vector c"=w488:dbl[])
        n257 = Negate(x=w479) -> (-x=w477:dbl[])
        n258 = Compound Arithmetic op=ADD(w479, w478, w488) -> (w486:dbl[])
        n259 = local read "Scale"() -> (w485:dbl)
        n260 = Divide(x=w486, y=2.0) -> (x/y=w484:dbl[])
        n261 = Multiply(x=w484, y=w485) -> (x*y=w483:dbl[])
        n262 = Multiply(x=w477, y=2.0 ("Numeric")) -> (x*y=w475:dbl[])
        n263 = Array To Cluster(array=w475) -> (cluster=w480:cluster{"[0]":dbl, "[1]":dbl, "[2]":dbl})
        n264 = Array To Cluster(array=w483) -> (cluster=w482:cluster{"[0]":dbl, "[1]":dbl, "[2]":dbl})
        n265 = Array To Cluster(array=w478) -> (cluster=w481:T26)
        n266 = invoke on="Invoke Node" class="SceneGraphDisp (strict)" method="Setup Camera"(reference=w474, "Camera Position"=w480, "Target"=w482, "Up Direction"=w481) -> ()  [unwired: 2 in, 6 out]
      }
      event "Make Awesome Looking": Value Change {
        n267 = event-data() -> ()  [unwired: 1 in, 4 out]
        n268 = control-ref of="Cd Rich Limit"() -> (w497:refnum<vi>)
        n269 = local read "Defect Energy Levels"() -> (w493:cluster{dbl[], dbl[]}[])
        n270 = local read "Cd Rich Limit"() -> (w495:cluster{"appended array":dbl[], dbl[]}[])
        n271 = local read "Te Rich Limit"() -> (w494:cluster{dbl[], dbl[]}[])
        n272 = property on="Defect Energy Levels" class="XYGraph (strict)"() -> ("AnntList"=w492:T27)  [unwired: 2 in, 2 out]
        n273 = Array Size(array=w495) -> (size(s)=w496:i32)
        n274 = for {
          N: w496 -> [_]
          tunnel: w497 -> [w513]
          tunnel: [w511] -> w490 mode=indexing
          tunnel: [w510] -> w491 mode=indexing
          i -> [w512]
          n275 = property on="Property Node" class="XYGraph (strict)"(reference=w513, "Active Plot"=w512) -> ("Plot.Plot Color"=w511:u32, "Plot.Plot Name"=w510:string)  [unwired: 1 in, 2 out]
        }
        n276 = disable-structure shown="Enabled" {
          disable-tunnel: w495 -> [w503 w505]
          disable-tunnel: w494 -> [w502 w506]
          disable-tunnel: w493 -> [w501 w507]
          disable-tunnel: w492 -> [w500 w509]
          disable-tunnel: w491 -> [w499 w504]
          disable-tunnel: w490 -> [w498 w508]
          frame Enabled {
            n277 = call "Awesome Looking Plots for Defect Buddy.vi"("Colors Array"=w498, "Plot Names"=w499, "Annotation List for Charge States"=w500, "Defect Energy Levels"=w501, "Te Rich Limit"=w502, "Cd Rich Limit"=w503) -> ()  [unwired: 6 in]
          }
          frame Disabled {
            n278 = call "Alter Plots for Presentations.vi"("Colors Array"=w508, "Plot Names"=w504, "Annotation List for Charge States"=w509, "Defect Energy Levels"=w507, "Te Rich Limit"=w506, "Cd Rich Limit"=w505) -> ()  [unwired: 6 in]
          }
        }
      }
    }
  }
  n279 = disable-structure shown="Disabled" {
    frame Disabled {
    }
    frame Enabled {
    }
  }
  n280 = disable-structure shown="Disabled" {
    frame Disabled {
      n281 = for {
        N: 9 -> [_]
        i -> [w523]
        n282 = control-ref of="Te Rich Limit"() -> (w517:refnum<vi>)
        n283 = property on="Property Node" class="XYGraph (strict)"(reference=w517, "Active Plot"=w523) -> ("Plot.Point Style"=w522:u8, "Plot.Fill/Pt. Color"=w521:u32, "Plot.Plot Color"=w520:u32, "Plot.Plot Interpolation"=w519:u8, "Plot.Line Width"=w518:u8, "Plot.Line Style"=w515:u8)  [unwired: 1 in, 2 out]
        n284 = control-ref of="Cd Rich Limit"() -> (w516:refnum<vi>)
        n285 = property on="Property Node" class="XYGraph (strict)"(reference=w516, "Active Plot"=w523, "Plot.Point Style"=w522, "Plot.Fill/Pt. Color"=w521, "Plot.Plot Color"=w520, "Plot.Plot Interpolation"=w519, "Plot.Line Width"=w518, "Plot.Line Style"=w515) -> ()  [unwired: 1 in, 2 out]
      }
    }
    frame Enabled {
    }
  }
